vi "GUI_Beampointing2_Pico.vi"() -> ()   [LabVIEW 2020]
uses:
  Shared/GUI_Template/GUI_master/tcp_new_data_event.ctl
  Shared/GUI_Template/GUI_master/tcp new data cluster.ctl
  Ctrs/beam detection.ctl
  Ctrs/move_old.ctl
  Ctrs/stats.ctl
  General GUIs/Device GUIs/GUI_Cameras/Controls/Crosshair type def.ctl
  Ctrs/Motor Calibration.ctl
  <vilib>/Analysis/NI_AALBase.lvlib
panel:
  out "Image":T1(plugin-control)
  in  "size 2":cluster{"xhair size":dbl, "xhair size 2":dbl}={"xhair size"=20.0, "xhair size 2"=20.0} {"xhair size 2" min=0.0 max=0.0; "xhair size" min=0.0 max=0.0}
  in  "Time":timestamp[](array[timestamp])
  in  "Stats 2":T2
  in  "output cluster 2":T3
  in  "UDP error message":string
  in  "Save Stats":bool
  in  "output cluster":T7={"img to avg"=0, "beam detection para"={"Filter"=0, "Filter Para"={"X Size"=0, "Y Size"=0, "% Tolerance"=0}, "detection method"=0, "smal para"=[], "Remove small Objects"=FALSE, "Restrict to round Objects"=FALSE}, "move"={"Tolerance [%]"=0.1, "Stepsize"=0.0001, "Invert Axis"=TRUE, "Invert Direction X"=FALSE, "Invert Direction Y"=TRUE, "enable feedback"=FALSE, "Set Centriod Target"=FALSE, "my active motor"=""}, "GUIdevice 1"="", "GUIdevice 2"="", "ActiveMotor"=0, "stats path "=path ""} {"beam detection para"."smal para"."Measurement Parameter" items=["Center of Mass X", "Center of Mass Y", "First Pixel X", "First Pixel Y", "Bounding Rect Left", "Bounding Rect Top", "Bounding Rect Right", "Bounding Rect Bottom", "Max Feret Diameter Start X", "Max Feret Diameter Start Y", "Max Feret Diameter End X", "Max Feret Diameter End Y", "Max Horiz. Segment Length Left", "Max Horiz. Segment Length Right", "Max Horiz. Segment Length Row", "-", "Bounding Rect Width", "Bounding Rect Height", "Bounding Rect Diagonal", "Perimeter", "Convex Hull Perimeter", "Holes' Perimeter", "Max Feret Diameter", "Equivalent Ellipse Major Axis", "Equivalent Ellipse Minor Axis", "Equivalent Ellipse Minor Axis (Feret)", "Equivalent Rect Long Side", "Equivalent Rect Short Side", "Equivalent Rect Diagonal", "Equivalent Rect Short Side (Feret)", "Average Horiz. Segment Length", "Average Vert. Segment Length", "Hydraulic Radius", "Waddel Disk Diameter", "-", "Area", "Holes' Area", "Particle & Holes' Area", "Convex Hull Area", "Image Area", "-", "Number of Holes", "Number of Horiz. Segments", "Number of Vert. Segments", "-", "Orientation", "Max Feret Diameter Orientation", "-", "% Area/Image Area", "% Area/(Particle & Holes' Area)", "Ratio of Equivalent Ellipse Axes", "Ratio of Equivalent Rect Sides", "-", "Elongation Factor", "Compactness Factor", "Heywood Circularity Factor", "Type Factor", "-", "Sum X", "Sum Y", "Sum XX", "Sum XY", "Sum YY", "Sum XXX", "Sum XXY", "Sum XYY", "Sum YYY", "-", "Moment of Inertia XX", "Moment of Inertia XY", "Moment of Inertia YY", "Moment of Inertia XXX", "Moment of Inertia XXY", "Moment of Inertia XYY", "Moment of Inertia YYY", "Norm. Moment of Inertia XX", "Norm. Moment of Inertia XY", "Norm. Moment of Inertia YY", "Norm. Moment of Inertia XXX", "Norm. Moment of Inertia XXY", "Norm. Moment of Inertia XYY", "Norm. Moment of Inertia YYY", "Hu Moment 1", "Hu Moment 2", "Hu Moment 3", "Hu Moment 4", "Hu Moment 5", "Hu Moment 6", "Hu Moment 7"]; "beam detection para"."smal para"."Range Lower Value" format="%.2f"; "beam detection para"."smal para"."Range Upper Value" format="%.2f"; "beam detection para"."detection method" items=["clustering", "entropy", "metric", "moments", "inter-class variance"]; "beam detection para"."Filter" items=["No Filter", "Median Filter", "Low Pass Filter"]}
  in  "Trigger::1":bool
  in  "Triggerdelay::1":dbl=0.003 min=0.0 max=50000.0 format="%#_6f"
  in  "Exposure::1":dbl=0.095 min=0.0001 max=1.0 format="%#_6f"
  in  "ActiveMotorName::2":string
  in  "RelativeSettings.Axis 1.StepSize::2":dbl=50.0 caption="Axis 1 Stepsize" min=0.0 max=999999.0 format="%_4p"
  in  "RelativeSettings.Axis 2.StepSize::2":dbl=50.0 caption="Axis 2 StepSize" min=0.0 max=999999.0 format="%_4p"
  in  "RelativeSettings.Axis 2.Position::2":dbl caption="Axis 2 Position" min=-999999.0 max=999999.0 format="%_4p"
  in  "RelativeSettings.Axis 1.Position::2":dbl caption="Axis 1 Position" min=-999999.0 max=999999.0 format="%_4p"
  in  "RelativeMove.Axis 2.CW::2":bool caption="RelativeMove.Axis 2.CW::1"
  in  "RelativeMove.Axis 2.CCW::2":bool caption="RelativeMove.Axis. 2.CCW::1"
  in  "RelativeMove.Axis 1.CW::2":bool caption="RelativeMove.Axis 1.CW::1"
  in  "RelativeMove.Axis 1.CCW::2":bool caption="RelativeMove.Axis 1.CCW::1"
  out "Names":string[](array[string])=["PA2_Input1", "PA2_Input2", "L2_TelInpFar", "L1_TelInpNear", "L4_TREXPASS1", "L5_TREXPass2", "L6_TREXPass3", "L7_TREXPass4", "L8_M10Leak", "B1_TelInput", "B2_TelLens1"]
  in  "ActiveMotor":u16(ring)=7 items=["PA2_Input1", "PA2_Input2", "L2_TelInpFar", "L1_TelInpNear"]
  in  "Set Centriod Target":bool
  in  "size":dbl=10.299999999999997
  in  "Tab Control 2":enum32{"CCD Original ", "CCD Detected"}(tab)=enum."CCD Detected"
  out "image::1":T1(plugin-control) caption="StagingM1Far"
  out "Beam":T1(plugin-control)
  in  "Reset History":bool
  out "centriod X":dbl[](graph)=[249.59745762711864, 249.9873417721519, 249.85593220338984]
  out "centriod Y":dbl[](graph)=[256.39830508474574, 256.0126582278481, 257.0]
  out "Stats":cluster{timestamp[], dbl[]}[](graph)
  in  "Tab Control":enum32{"System", "Detection", "Feedback"}(tab)=enum."Feedback"
  in  "Save Stats":bool
  in  "update speed [ms]":i32=200
  in  "img to avg":i32=20
  in  "Save Config":bool
  in  "Load Config":bool
  in  "Cameras":u16(ring)=15 items=["10TW_Driver_Spot_Cam", "B1_TelInput", "B2_TelLens1", "B3_TelLens2", "B5_CompressorOut", "B6_SwitchYNear", "B9_OAPFront", "GIGEtest", "L1_TelInpNear", "L2_TelInpFar", "L3_TelescopeOut", "L4_TREXpass1", "L5_TREXPass2", "L6_TREXpass3", "L7_TREXPass4", "L8_M10Leak", "OAPtestCam", "PA2_Input1", "PA2_Input2", "PaperCam", "StagingAlignBeam1", "StagingAlignBeam2", "StagingCapAlignment", "StagingCapSpec", "StagingCapSpec1stOrder", "StagingChromaxGuppy", "StagingDiodeMonitor", "StagingFocusBeam1", "StagingFocusBeam2", "StagingGuppy", "StagingM1Far", "StagingM1Near", "StagingM3Far", "StagingM4", "StagingM5", "StagingMagnetCam1", "StagingMagnetCam2", "StagingMagnetCam3", "StagingManta2", "StagingModeImager2", "StagingModeTemp", "StagingOAP1Far", "StagingOAP1Near", "StagingOAP2Far", "StagingOAP2Near", "StagingPhasics", "StagingPhosphor", "StagingTapeCam", "StagingTapeMonitorCam", "StagingTopView", "TargetCam10Hz_Diode", "TargetCam1Hz_Pulsed", "TREXVarianCam0", "TREXVarianCam1", "TREXVarianCam2", "TREXVarianCam3", "TREX_CapSideView", "TREX_TA6", "TS-253a_in", "TS-CapSideview", "TS-CapSpec", "TS-ChromexCam", "TS-InputNearField", "TS-Mode1", "TS-OverlapCam", "TS-Periscope", "XUV_Cam1", "XUV_Cam2"]
  in  "calibrate":bool
  in  "stats path":path
  in  "beam detection para":T4={"Filter"=1, "Filter Para"={"X Size"=5, "Y Size"=5, "% Tolerance"=1}, "detection method"=4, "smal para"=[{"Measurement Parameter"=35, "Range Lower Value"=150.0, "Range Upper Value"=300.0, "Range"=FALSE, "Measurement Type"=FALSE}], "Remove small Objects"=TRUE, "Restrict to round Objects"=FALSE} {"smal para"."Measurement Parameter" items=["Center of Mass X", "Center of Mass Y", "First Pixel X", "First Pixel Y", "Bounding Rect Left", "Bounding Rect Top", "Bounding Rect Right", "Bounding Rect Bottom", "Max Feret Diameter Start X", "Max Feret Diameter Start Y", "Max Feret Diameter End X", "Max Feret Diameter End Y", "Max Horiz. Segment Length Left", "Max Horiz. Segment Length Right", "Max Horiz. Segment Length Row", "-", "Bounding Rect Width", "Bounding Rect Height", "Bounding Rect Diagonal", "Perimeter", "Convex Hull Perimeter", "Holes' Perimeter", "Max Feret Diameter", "Equivalent Ellipse Major Axis", "Equivalent Ellipse Minor Axis", "Equivalent Ellipse Minor Axis (Feret)", "Equivalent Rect Long Side", "Equivalent Rect Short Side", "Equivalent Rect Diagonal", "Equivalent Rect Short Side (Feret)", "Average Horiz. Segment Length", "Average Vert. Segment Length", "Hydraulic Radius", "Waddel Disk Diameter", "-", "Area", "Holes' Area", "Particle & Holes' Area", "Convex Hull Area", "Image Area", "-", "Number of Holes", "Number of Horiz. Segments", "Number of Vert. Segments", "-", "Orientation", "Max Feret Diameter Orientation", "-", "% Area/Image Area", "% Area/(Particle & Holes' Area)", "Ratio of Equivalent Ellipse Axes", "Ratio of Equivalent Rect Sides", "-", "Elongation Factor", "Compactness Factor", "Heywood Circularity Factor", "Type Factor", "-", "Sum X", "Sum Y", "Sum XX", "Sum XY", "Sum YY", "Sum XXX", "Sum XXY", "Sum XYY", "Sum YYY", "-", "Moment of Inertia XX", "Moment of Inertia XY", "Moment of Inertia YY", "Moment of Inertia XXX", "Moment of Inertia XXY", "Moment of Inertia XYY", "Moment of Inertia YYY", "Norm. Moment of Inertia XX", "Norm. Moment of Inertia XY", "Norm. Moment of Inertia YY", "Norm. Moment of Inertia XXX", "Norm. Moment of Inertia XXY", "Norm. Moment of Inertia XYY", "Norm. Moment of Inertia YYY", "Hu Moment 1", "Hu Moment 2", "Hu Moment 3", "Hu Moment 4", "Hu Moment 5", "Hu Moment 6", "Hu Moment 7"]; "smal para"."Range Lower Value" format="%.2f"; "smal para"."Range Upper Value" format="%.2f"; "detection method" items=["clustering", "entropy", "metric", "moments", "inter-class variance"]; "Filter" items=["No Filter", "Median Filter", "Low Pass Filter"]}
  in  "Move Properties":T6={"Tolerance [%]"=0.1, "Stepsize"=0.0001, "Invert Axis"=TRUE, "Invert Direction X"=FALSE, "Invert Direction Y"=TRUE, "enable feedback"=FALSE, "Set Centriod Target"=FALSE, "my active motor"=""} {"Stepsize" format="%#_6p"}
  out "Y Size":dbl=20.599999999999994
  out "X Size":dbl=15.599999999999994
  out "Particle Reports (Pixels)":T8(array[cluster])=[{"Area"=236.0, "Number of Holes"=0.0, "Bounding Rect"={"Left"=243.0, "Top"=247.0, "Right"=258.0, "Bottom"=268.0}, "Center of Mass"={"X"=249.85593220338984, "Y"=257.0}, "Orientation"=87.89795034558499, "Dimensions"={"Width"=15.0, "Height"=21.0}}] {"Orientation" format="%.2f"; "Dimensions"."Height" format="%.2f"; "Dimensions"."Width" format="%.2f"; "Center of Mass"."Y" format="%.2f"; "Center of Mass"."X" format="%.2f"; "Bounding Rect"."Bottom" format="%.2f"; "Bounding Rect"."Right" format="%.2f"; "Bounding Rect"."Top" format="%.2f"; "Bounding Rect"."Left" format="%.2f"; "Number of Holes" format="%.2f"; "Area" format="%.2f"}
  out "move required":bool=TRUE
  out "moving":bool
  out "Best Rectangle":T9(array[cluster])=[{"Left"=243.0, "Top"=247.0, "Right"=259.0, "Bottom"=267.0}, {"Left"=242.0, "Top"=246.0, "Right"=257.0, "Bottom"=267.0}, {"Left"=242.0, "Top"=246.0, "Right"=258.0, "Bottom"=267.0}, {"Left"=243.0, "Top"=247.0, "Right"=258.0, "Bottom"=268.0}, {"Left"=242.0, "Top"=247.0, "Right"=258.0, "Bottom"=267.0}]
  out "XY Graph":cluster{timestamp[], dbl[]}[](graph)
  out "Y offset":dbl=-1.5635377104373447
  out "X offset":dbl=10.405838585398385
  in  "Target.X::1":dbl=260.0 min=0.0 max=2000.0 format="%#_6f"
  in  "Target.Y::1":dbl=255.0 min=0.0 max=2000.0 format="%#_6f"
  out "mean Y":dbl=256.56353771043734 format="%0.2f"
  out "mean X":dbl=249.59416141460161 format="%0.2f"
  out "beam detected":bool=TRUE
  in  "GUIdevice 2":string="Picopad4"
  out "error out":errorcluster
  in  "insert tag":bool=TRUE
  in  "stop":bool=TRUE
  in  "GUIdevice 1":string="B5_CompressorOut"
  out "tcp data event":T10
  out "error IO 2":errorcluster
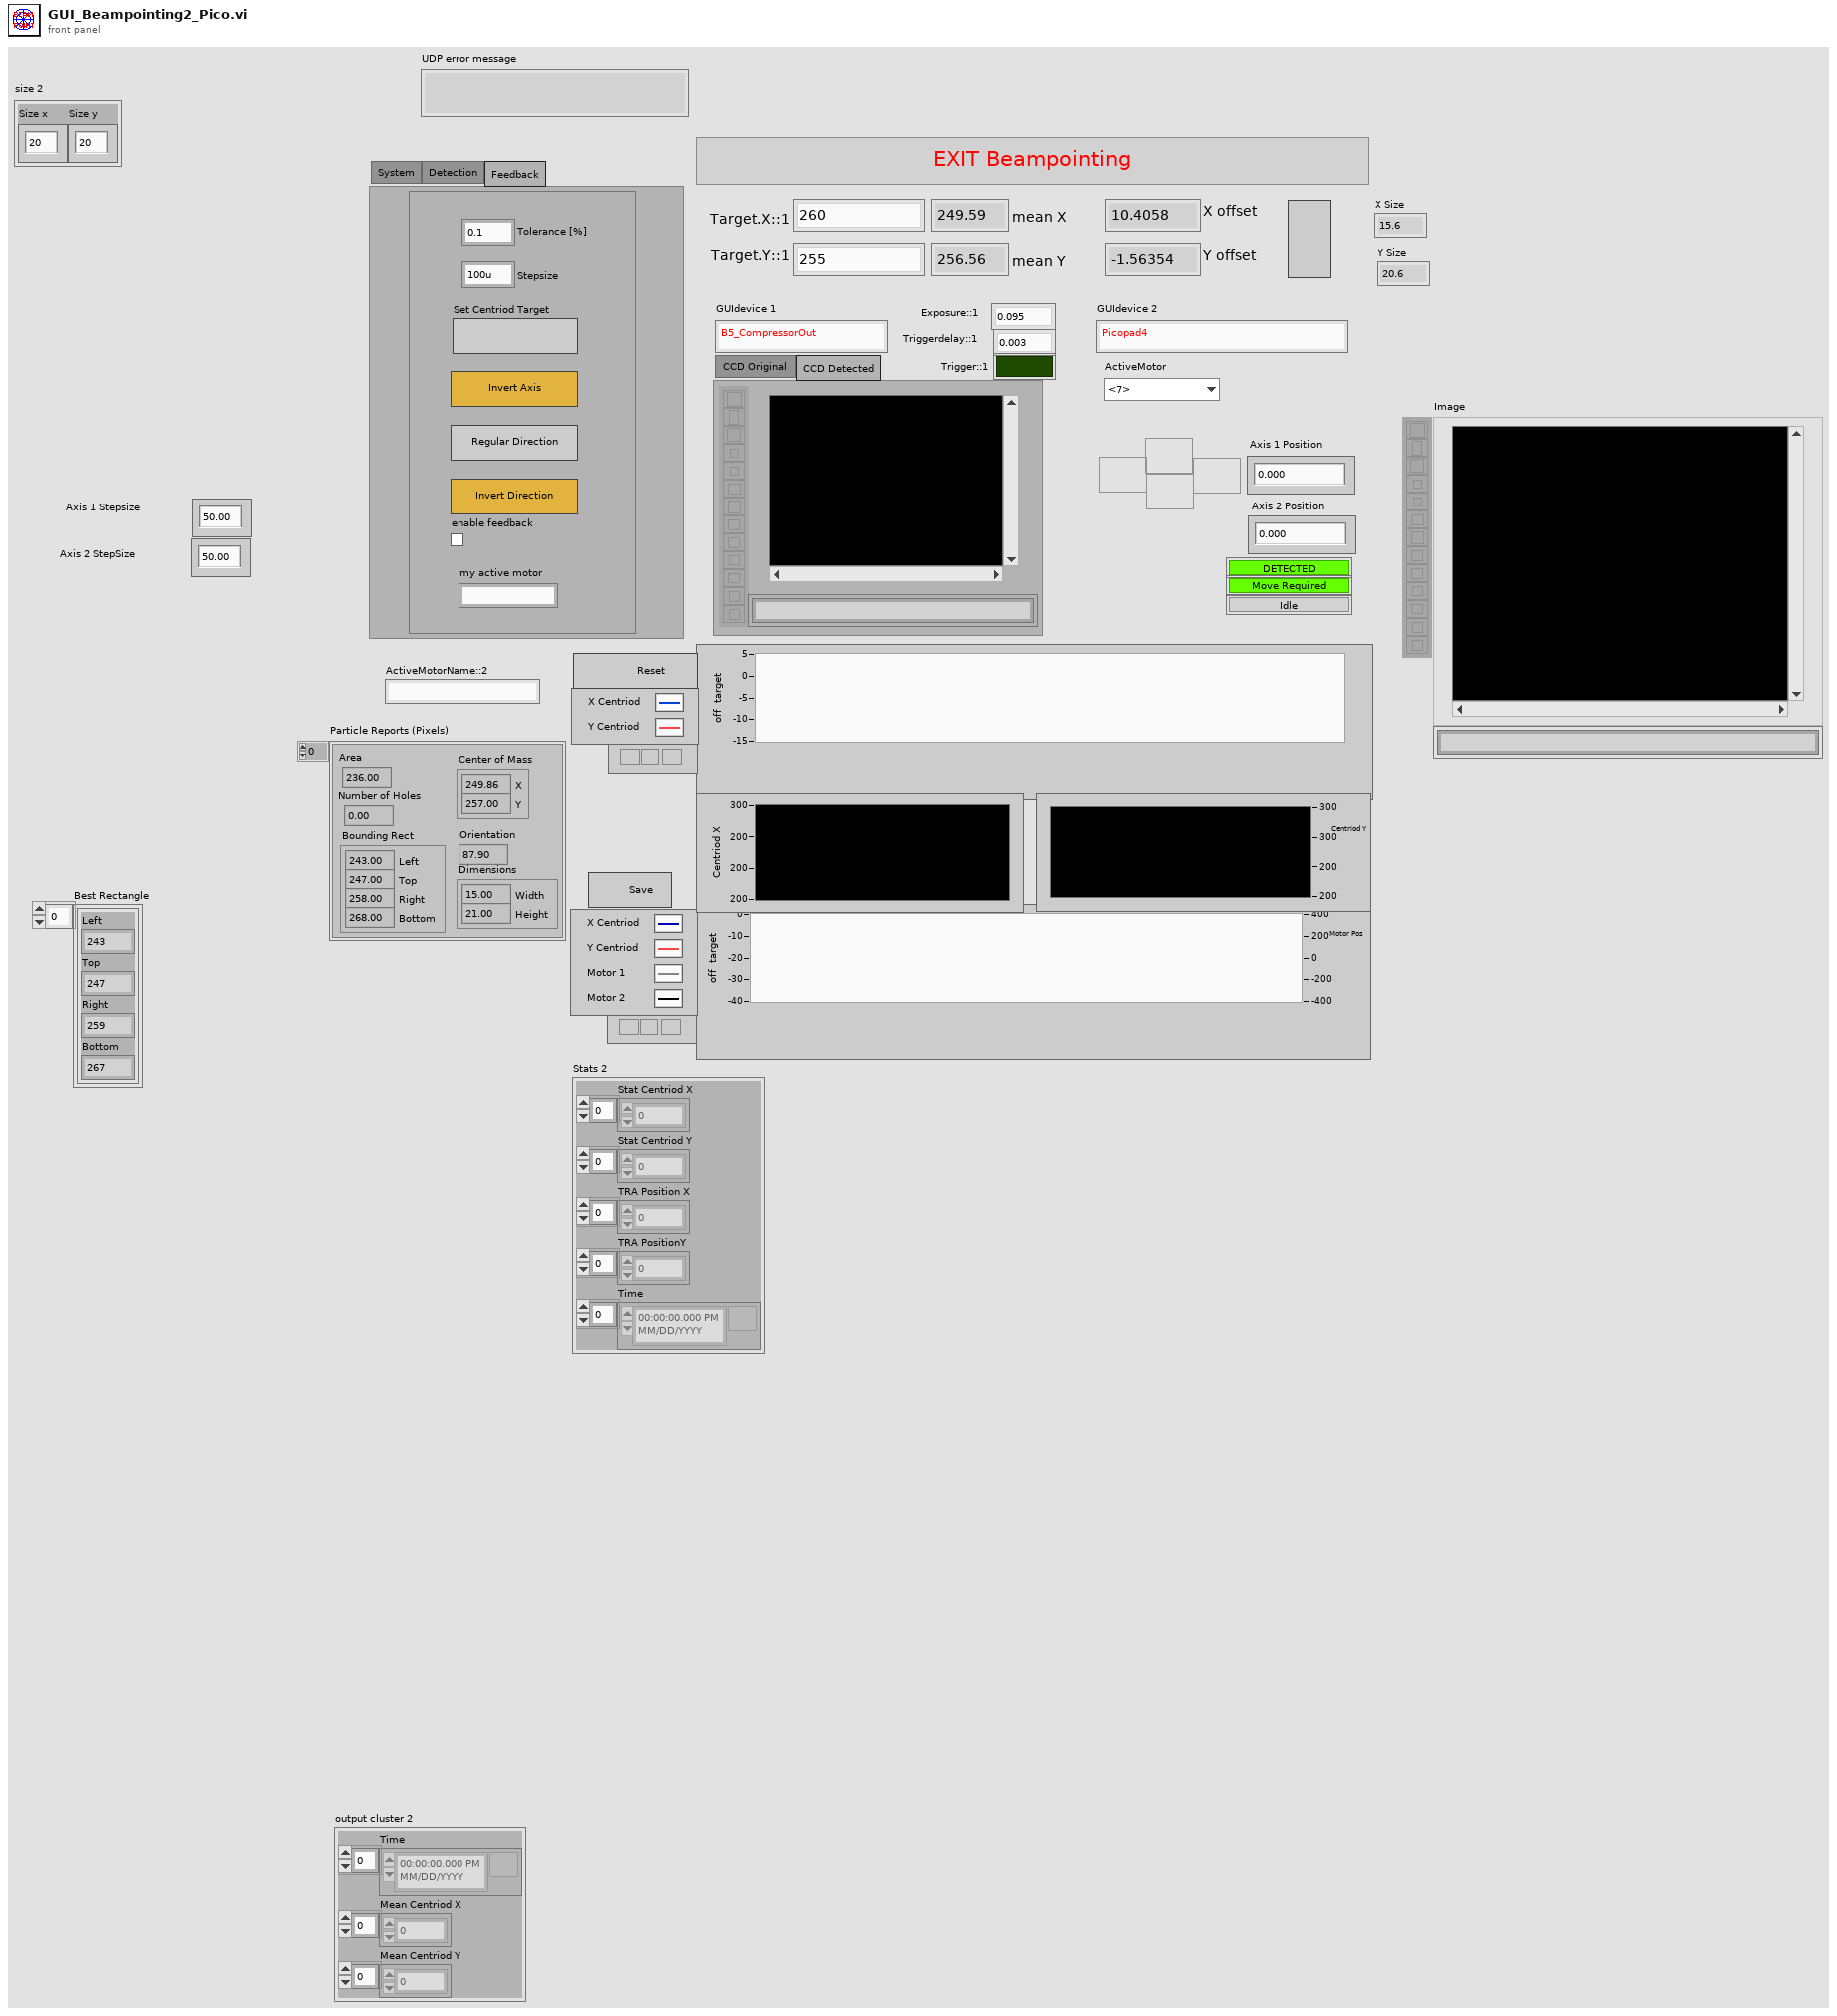
[diagram p1: front panel]
types:
  T1 = typedef "IMAQ Image.ctl" = refnum<image>
  T2 = typedef "stats.ctl" = cluster{"Stat Centriod X":dbl[], "Stat Centriod Y":dbl[], "TRA Position X":dbl[], "TRA PositionY":dbl[], "Time":timestamp[]}
  T3 = cluster{"Time":timestamp[], "Mean Centriod X":dbl[], "Mean Centriod Y":dbl[]}
  T4 = typedef "beam detection.ctl" = cluster{"Filter":u16, "Filter Para":cluster{"X Size":i32, "Y Size":i32, "% Tolerance":i32}, "detection method":i32, "smal para":cluster{"Measurement Parameter":T5, "Range Lower Value":dbl, "Range Upper Value":dbl, "Range":bool, "Measurement Type":bool}[], "Remove small Objects":bool, "Restrict to round Objects":bool}
  T5 = typedef "Particle Parameters" = i32
  T6 = typedef "move_old.ctl" = cluster{"Tolerance [%]":dbl, "Stepsize":dbl, "Invert Axis":bool, "Invert Direction X":bool, "Invert Direction Y":bool, "enable feedback":bool, "Set Centriod Target":bool, "my active motor":string}
  T7 = cluster{"img to avg":i32, "beam detection para":T4, "move":T6, "GUIdevice 1":string, "GUIdevice 2":string, "ActiveMotor":u16, "stats path ":path}
  T8 = cluster{"Area":dbl, "Number of Holes":dbl, "Bounding Rect":cluster{"Left":dbl, "Top":dbl, "Right":dbl, "Bottom":dbl}, "Center of Mass":cluster{"X":dbl, "Y":dbl}, "Orientation":dbl, "Dimensions":cluster{"Width":dbl, "Height":dbl}}[]
  T9 = cluster{"Left":dbl, "Top":dbl, "Right":dbl, "Bottom":dbl}[]
  T10 = typedef "tcp_new_data_event.ctl" = refnum<user-event>
  T11 = typedef "tcp new data cluster.ctl" = cluster{"EventEnum":enum16{"new data", "connection status update"}, "Device name":string}
  T12 = typedef "Image Type" = u32
  T13 = cluster{"RelativeMove.Axis 1.CW::2":refnum<vi>, "RelativeMove.Axis 1.CCW::2":refnum<vi>, "RelativeMove.Axis 2.CW::2":refnum<vi>, "RelativeMove.Axis 2.CCW::2":refnum<vi>}
  T14 = typedef "Crosshair type def.ctl" = cluster{"Draw":bool, "Target":cluster{"x":dbl, "y":dbl}, "Size":cluster{"x":dbl, "y":dbl}, "Angle":dbl, "Color":u32, "Thickness":u8, "CrosshairLabel":string}
  T15 = cluster{"Left":i32, "Top":i32, "Right":i32, "Bottom":i32}
  T16 = enum32{"invalid app kind", "Development System", "Run Time System", "Student Edition", "Embedded LabVIEW", "Evaluation", "Custom"}
  T17 = enum32{"Invalid", "Standard", "Closed", "Hidden", "Minimized", "Maximized"}
  T18 = enum16{"open", "replace", "create", "open or create", "replace or create", "replace or create with confirmation"}
  T19 = typedef "Motor Calibration.ctl" = cluster{"Slope Axis 1":dbl, "Axis Inverted":bool, "Slope Axis 2":dbl, "Axis 1 revered":bool, "Axis 2 revered":bool}
  T20 = cluster{"Core":cluster{"Current VI Reference":refnum<vi>, "Close Panel on Exit?":bool}, "beam detection para":T4, "Centriod X":dbl[], "Centriod Y":dbl[], "Best Rectangle":cluster{"Left":dbl, "Top":dbl, "Right":dbl, "Bottom":dbl}[], "PArticle Report":cluster{"Area":dbl, "Number of Holes":dbl, "Bounding Rect":cluster{"Left":dbl, "Top":dbl, "Right":dbl, "Bottom":dbl}, "Center of Mass":cluster{"X":dbl, "Y":dbl}, "Orientation":dbl, "Dimensions":cluster{"Width":dbl, "Height":dbl}}[], "Mean Centriod X":dbl[], "Mean Centriod Y":dbl[], "Time":timestamp[], "beam detected":bool, "offsets":cluster{"X offset":dbl, "Y offset":dbl}, "move":T6, "moving":bool, "Stats":T2, "set centriod target":bool, "Motor Calibration":T19}
  T21 = cluster{"Left":dbl, "Top":dbl, "Right":dbl, "Bottom":dbl}
  T22 = cluster{"Current VI Reference":refnum<vi>, "Close Panel on Exit?":bool}
  T23 = cluster{"Time":timestamp[], "Stat Centriod X":dbl[]}
  T24 = cluster{"Time":timestamp[], "Stat Centriod Y":dbl[]}
  T25 = cluster{"Time":timestamp[], "TRA Position X":dbl[]}
  T26 = cluster{"Time":timestamp[], "TRA PositionY":dbl[]}
  T27 = cluster{"Time":timestamp[], "TRA PositionY":dbl[]}[]
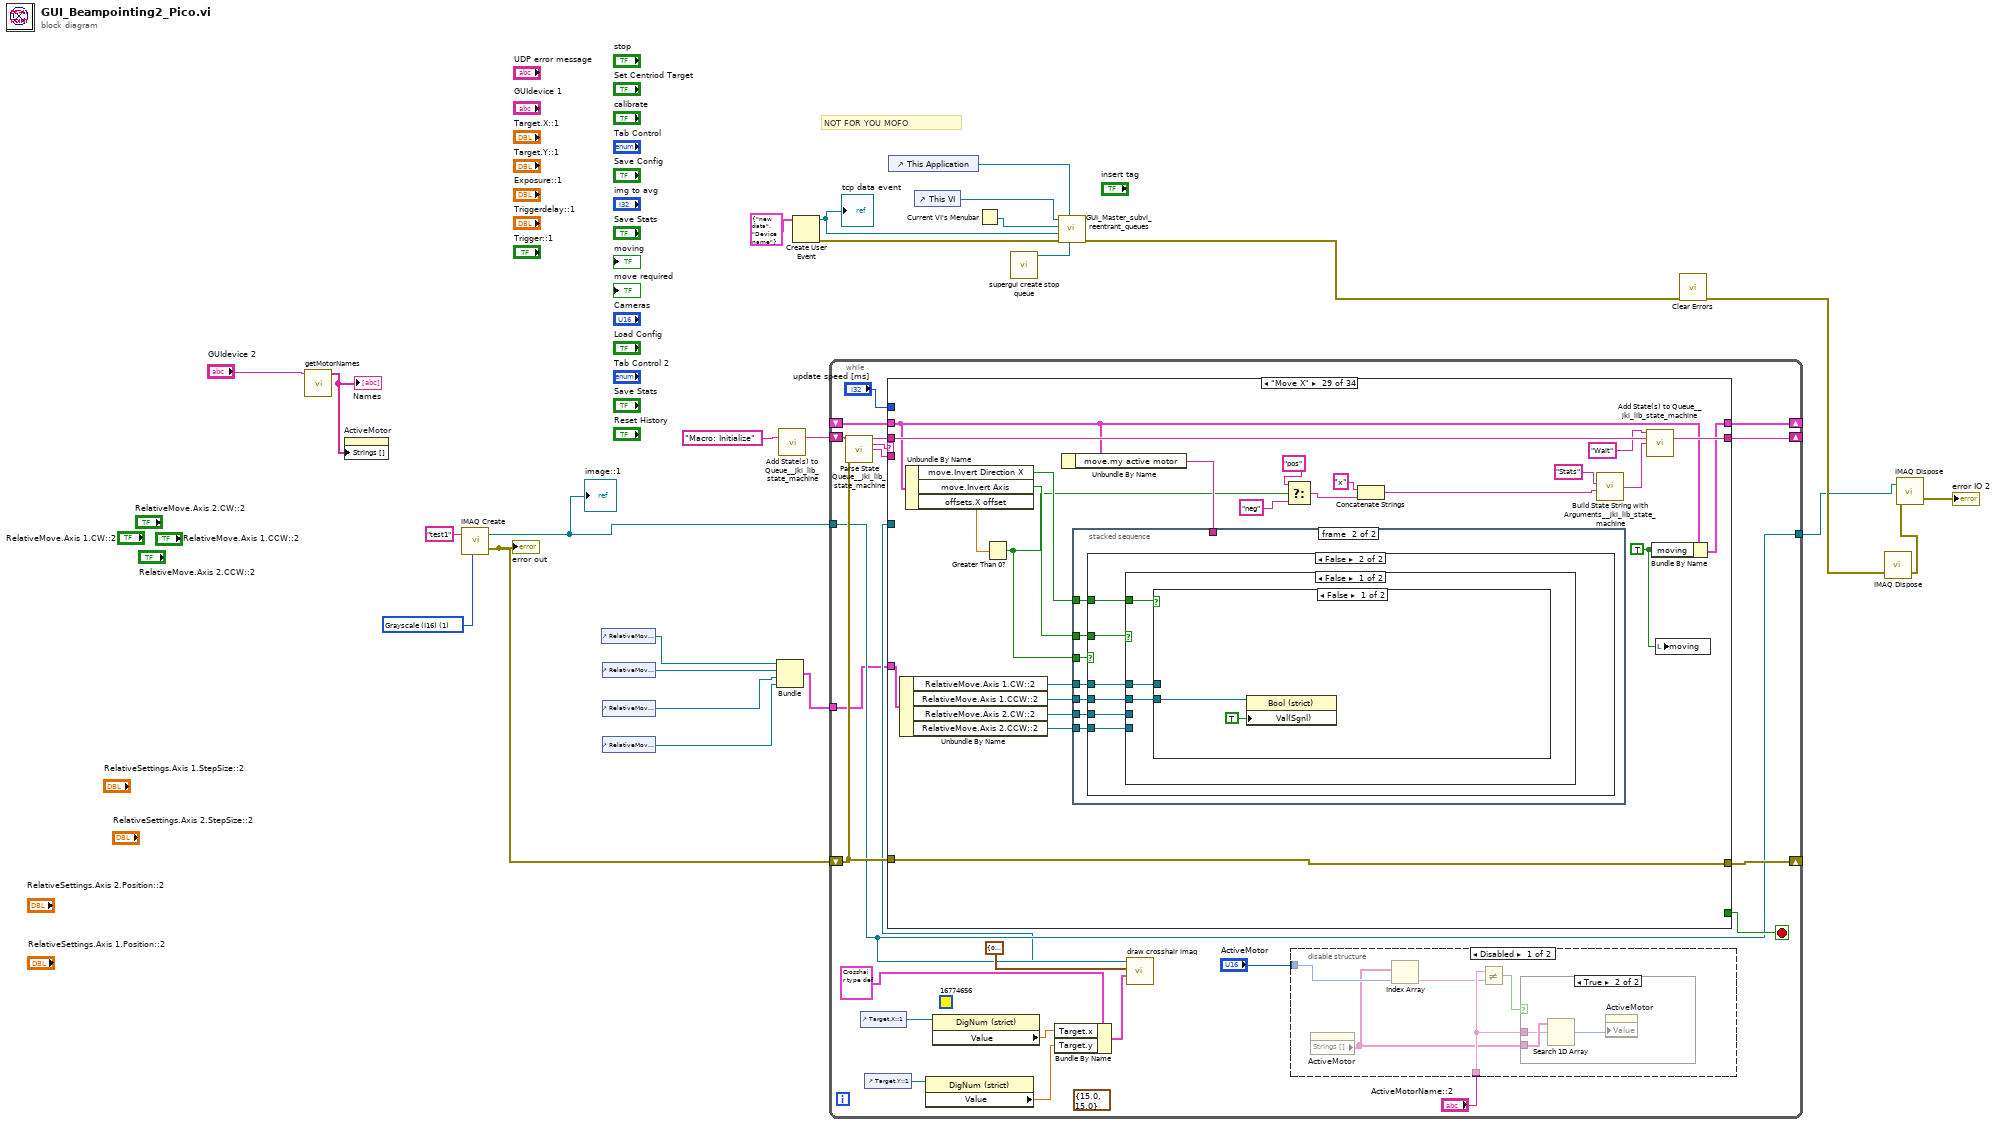
[diagram p0: block diagram]
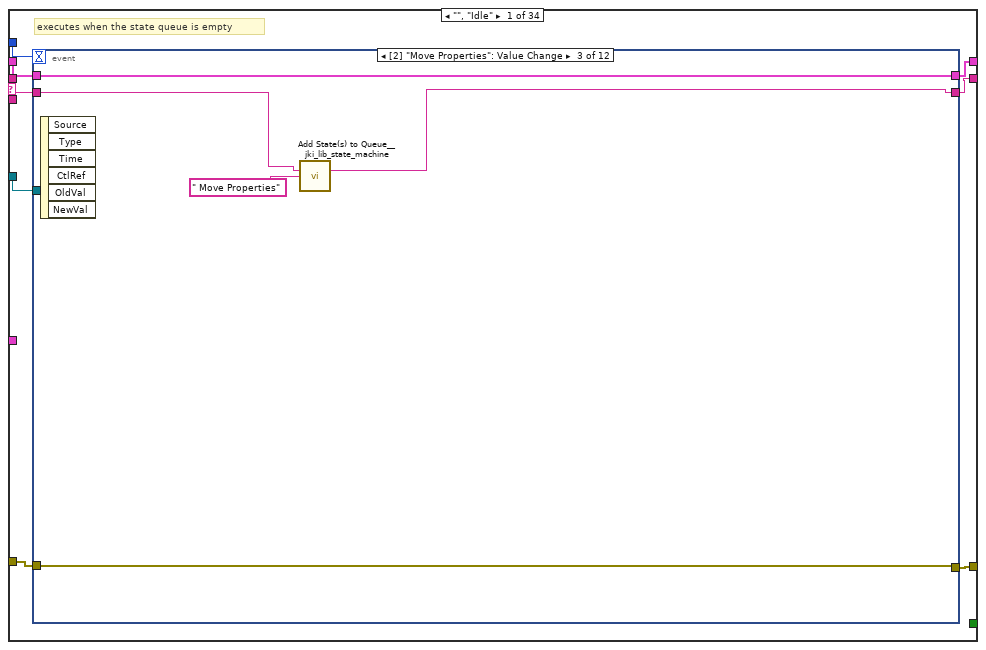
[diagram p4: hidden frame]
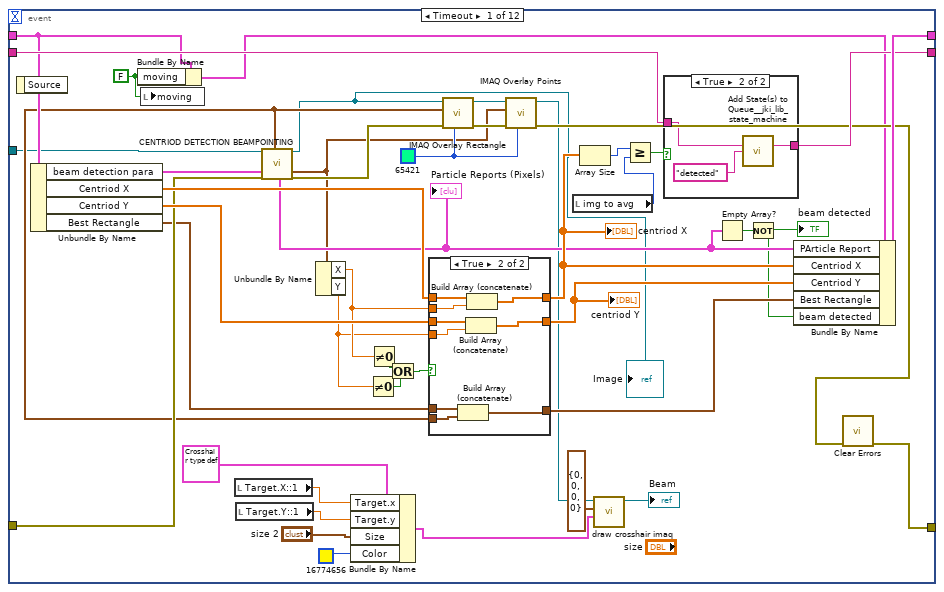
[diagram p5: hidden frame]
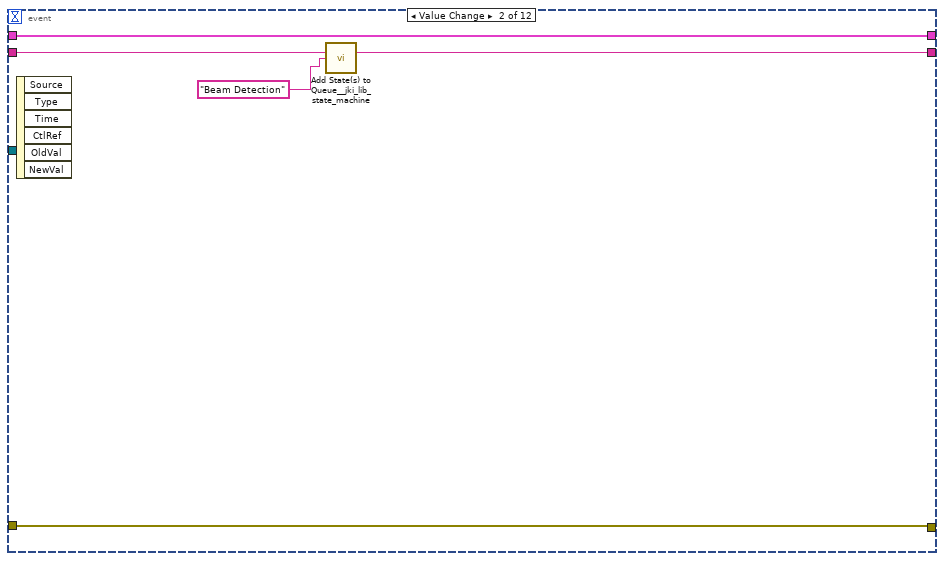
[diagram p8: hidden frame]
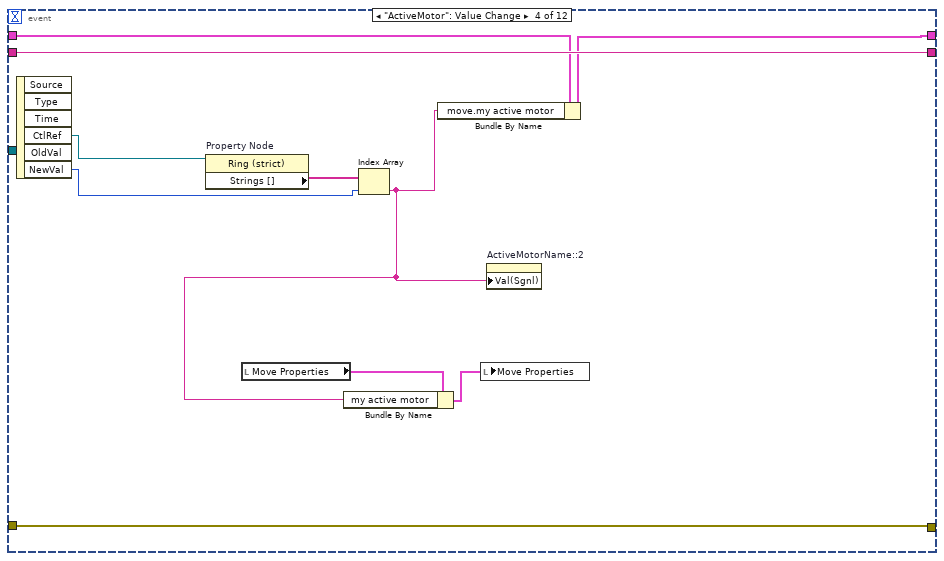
[diagram p9: hidden frame]
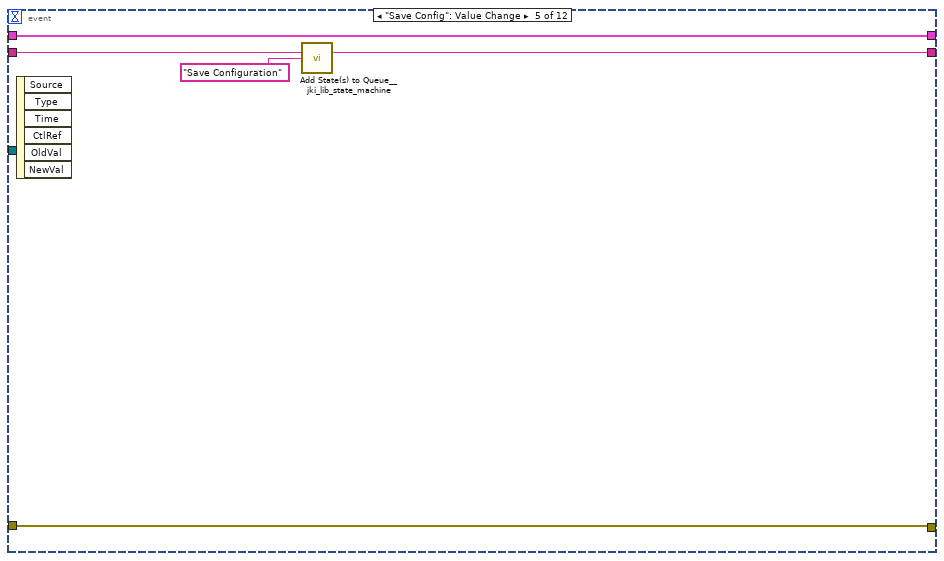
[diagram p10: hidden frame]
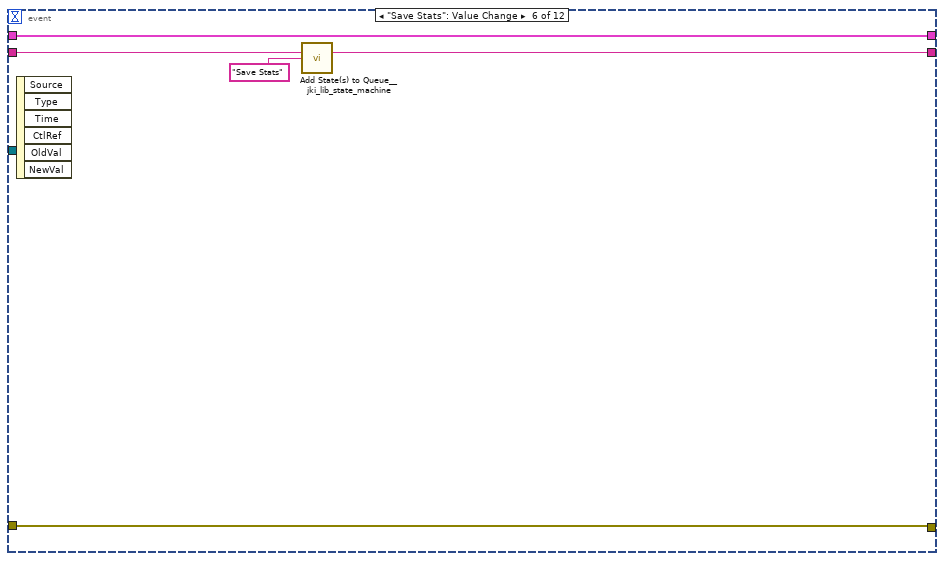
[diagram p11: hidden frame]
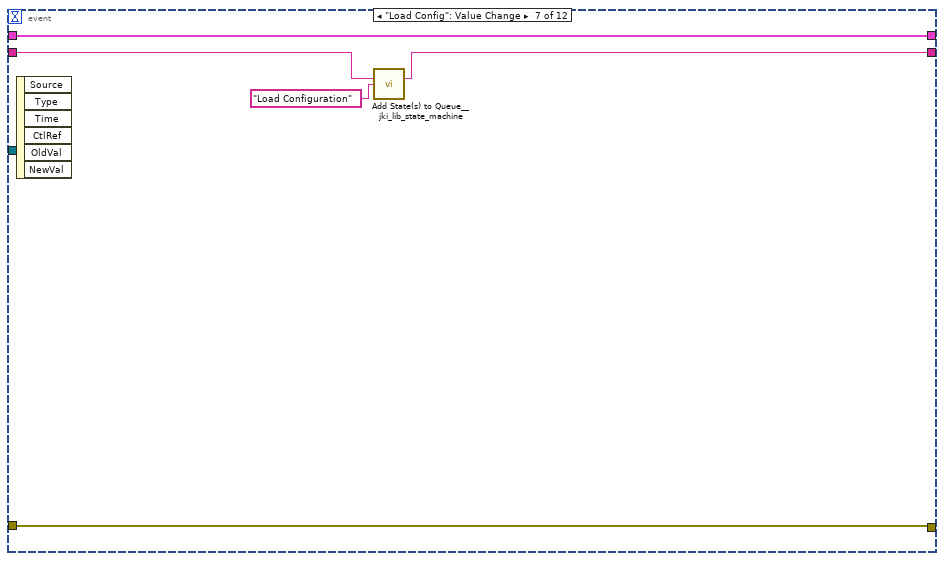
[diagram p12: hidden frame]
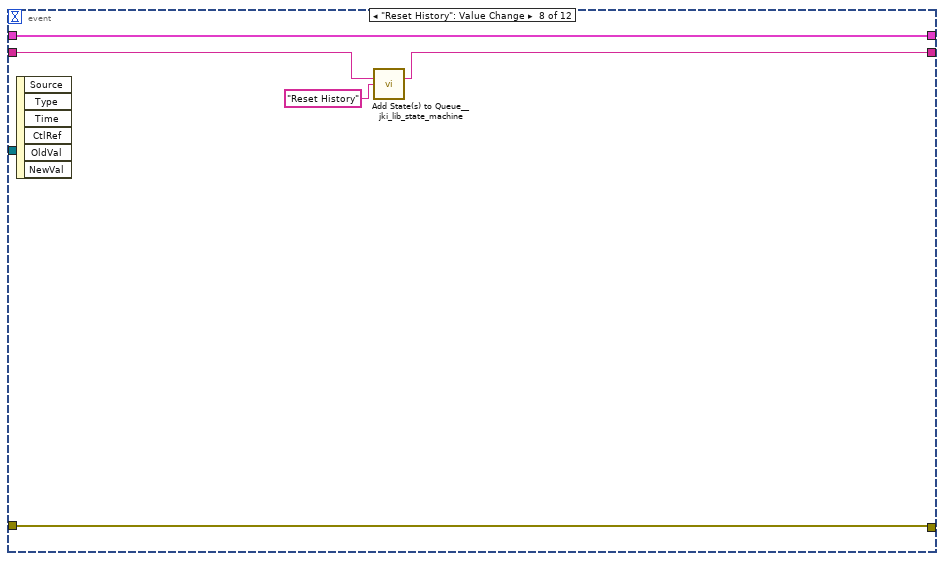
[diagram p13: hidden frame]
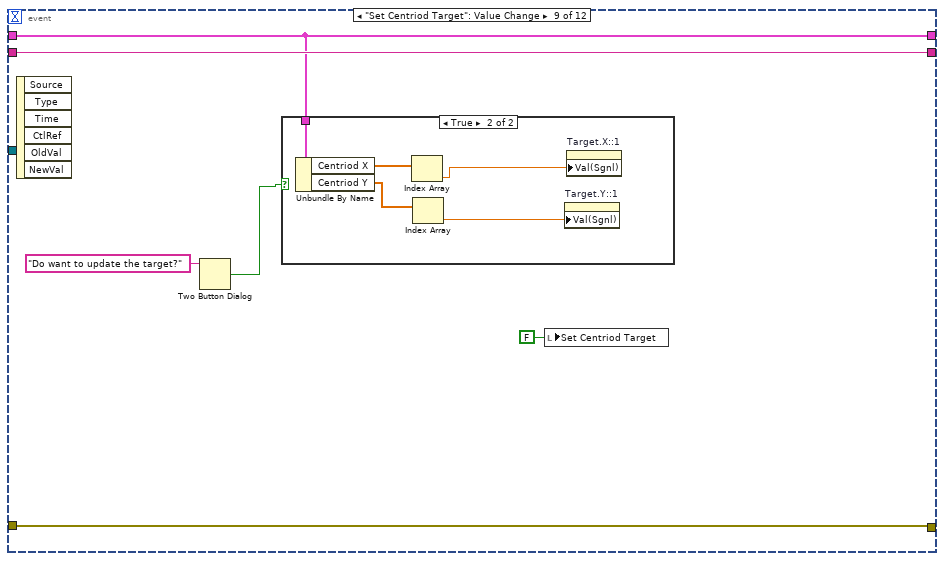
[diagram p14: hidden frame]
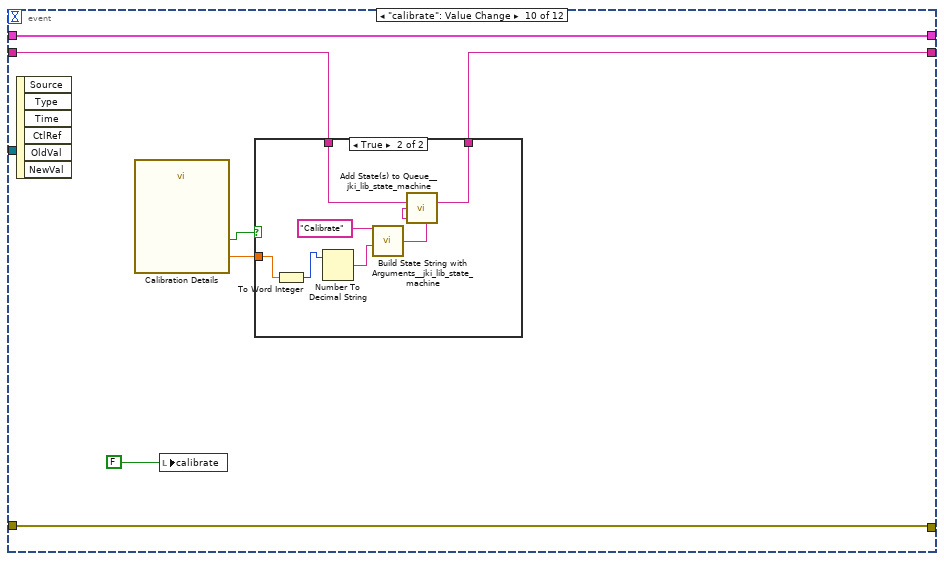
[diagram p16: hidden frame]
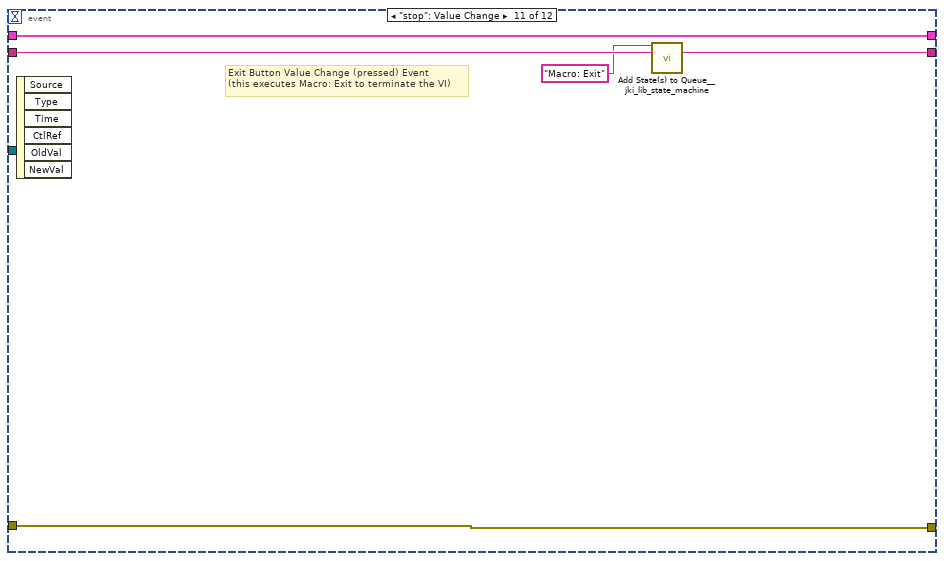
[diagram p18: hidden frame]
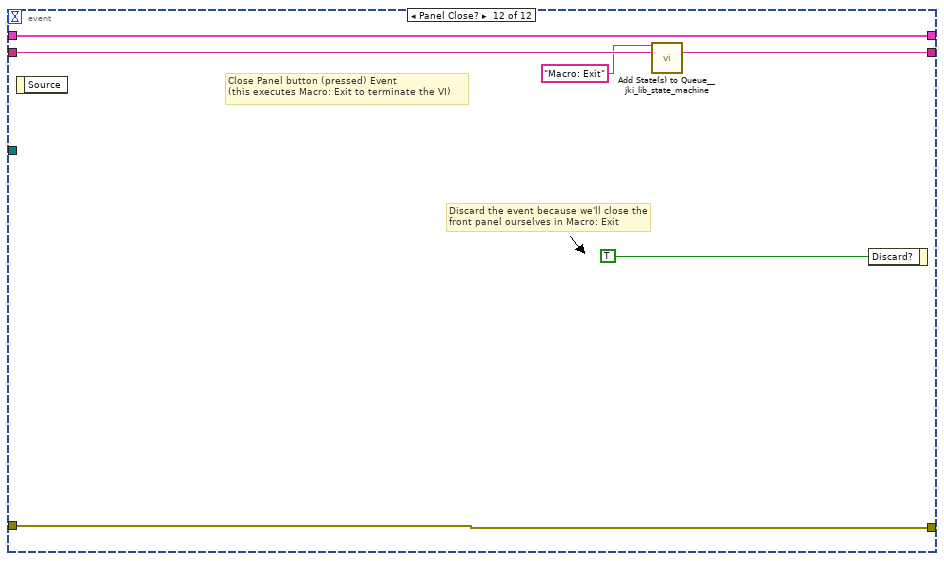
[diagram p19: hidden frame]
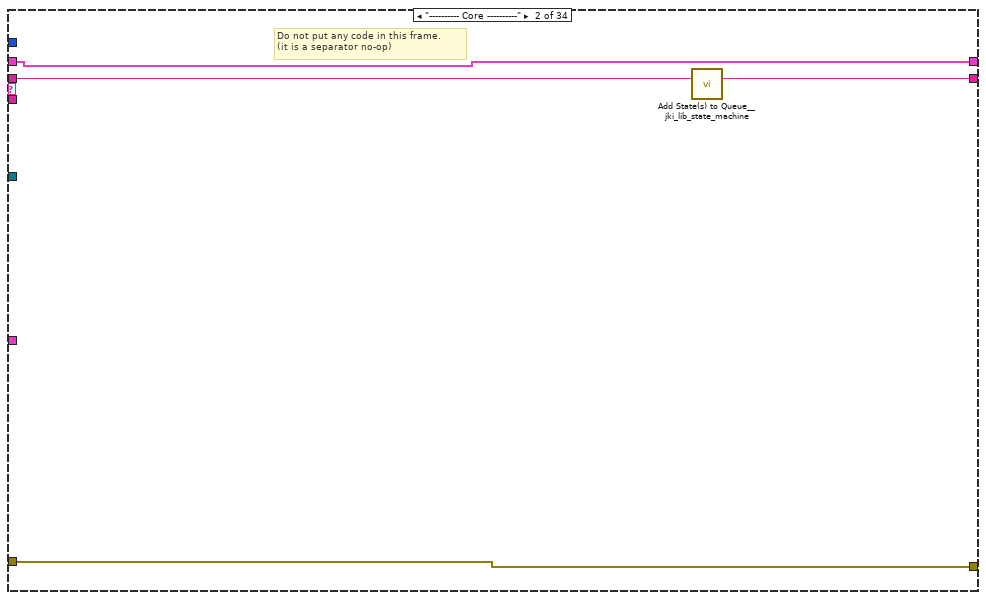
[diagram p20: hidden frame]
diagram:
  w24 = T12 1 items=["Grayscale (U8)", "Grayscale (I16)", "Grayscale (SGL)", "Complex (CSG)", "RGB (U32)", "HSL (U32)", "RGB (U64)", "Grayscale (U16)"] ("Image Type")
  # "NOT FOR YOU MOFO"
  n1 = call "getMotorNames.vi"("DeviceName"="GUIdevice 2") -> ("elements"=w7:string[])  [unwired: 10 in]
  "Names" <- w7
  n2 = property on="ActiveMotor" class="Ring (strict)"("Strings []"=w7) -> ()  [unwired: 2 in, 2 out]
  n3 = call "IMAQ Create"("Image Name"="test1", "Image Type"=w24) -> ("New Image"=w9:T1, "error out"=w17:errorcluster)  [unwired: 3 in]
  "error out" <- w17
  "image::1" <- w9
  n4 = control-ref of="RelativeMove.Axis 1.CW::2"() -> (w6:refnum<vi>)
  n5 = control-ref of="RelativeMove.Axis 1.CCW::2"() -> (w5:refnum<vi>)
  n6 = control-ref of="RelativeMove.Axis 2.CW::2"() -> (w4:refnum<vi>)
  n7 = control-ref of="RelativeMove.Axis 2.CCW::2"() -> (w3:refnum<vi>)
  n8 = Bundle("RelativeMove.Axis 1.CW::2"=w6, "RelativeMove.Axis 1.CCW::2"=w5, "RelativeMove.Axis 2.CW::2"=w4, "RelativeMove.Axis 2.CCW::2"=w3) -> (w2:T13)  [unwired: 1 in]
  n9 = call <vilib>:"Add State(s) to Queue__jki_lib_state_machine.vi"("State(s) in (\"\")"="Macro: Initialize") -> ("States Out"=w19:string)  [unwired: 14 in]
  n10 = Create User Event(user event datatype=T11 {"EventEnum"=enum."new data", "Device name"="Device name"} ("New Event")) -> (user event=w10:refnum<user-event>, error out=w12:errorcluster)  [unwired: 1 in]
  "tcp data event" <- w10
  n11 = while "JKI - String-Based Queued State Machine (Basic) v1.0" {
    shift-right: [w42] -> _
    shift-left: _ -> [w41]
    shift-right: [w44] -> _
    shift-left: w17 -> [w39]
    shift-right: [w43] -> _
    shift-left: w19 -> [w45]
    tunnel: w9 -> [w34]
    tunnel: [w34] -> w16
    tunnel: w2 -> [w32]
    stop <- w38 stop-if-true
    (unwired) cluster{"xhair size":dbl, "xhair size 2":dbl} {"xhair size"=15.0, "xhair size 2"=15.0} ("size")
    (unwired) u32 16774656 ("Color")
    n12 = call <vilib>:"Parse State Queue__jki_lib_state_machine.vi"("State Queue"=w45, "Error In (no error)"=w39) -> ("Remaining States"=w47:string, "Current State"=w48:string, "Arguments"=w46:string)  [unwired: 11 in]
    n13 = control-ref of="Target.X::1"() -> (w36:refnum<vi>)
    n14 = control-ref of="Target.Y::1"() -> (w37:refnum<vi>)
    n15 = property class="DigNum (strict)"(reference=w37) -> ("Value"=w27:dbl)  [unwired: 1 in, 2 out]
    n16 = property class="DigNum (strict)"(reference=w36) -> ("Value"=w28:dbl)  [unwired: 1 in, 2 out]
    n17 = Bundle By Name(cluster=T14 {"Draw"=TRUE, "Target"={"x"=25.0, "y"=25.0}, "Size"={"x"=25.0, "y"=25.0}, "Angle"=0.0, "Color"=8322834, "Thickness"=1, "CrosshairLabel"=""} ("Crosshair"), "Target.x"=w28, "Target.y"=w27) -> (w26:T14)
    n18 = call "draw crosshair imaq.vi"("Crosshair"=w26, "Bounding Rectangle"=T15 {"Left"=0, "Top"=0, "Right"=0, "Bottom"=0}, "image in"=w34) -> ("image out"=w33:T1)  [unwired: 7 in, 1 out]
    n19 = case shown="\"Move X\"" w48 {
      selector: w48 -> [_ _ w206 _ _ _ _ _ _ _ _ _ _ _ _ _ _ _ _ _ _ _ _ _ _ _ _ _ _ _ _ _ _ _]
      tunnel: w47 -> [w64 w205 w210 w228 w234 w239 w243 w267 w273 w277 w281 w287 w298 w324 w329 w339 w343 w349 w356 w377 w385 w406 w442 w450 w454 w487 w497 w534 w558 w630 w690 w703 w778 w782]
      tunnel: w46 -> [_ _ _ _ _ _ _ _ _ _ _ w282 w292 _ _ _ _ _ _ _ _ _ _ _ _ _ _ _ _ _ _ w696 w773 _]
      tunnel: w41 -> [w62 w202 w208 w219 w231 w237 w240 _ w269 w274 w279 w285 w294 w321 w326 w336 w340 w345 w352 w360 w383 w404 w434 w446 w451 w470 w499 w531 w545 w617 w686 w725 w775 w779]
      tunnel: [w61 w203 w212 w225 errorcluster {"status"=FALSE, "code"=0, "source"=""} ("error out") w236 w241 w264 w270 w275 w278 w283 w295 w322 w327 w337 w341 w347 w354 w365 w381 w402 w431 w448 w452 w486 w518 w532 w556 w628 w679 w727 w774 w780] -> w44
      tunnel: w39 -> [w60 w203 w211 w225 w230 w236 w241 w264 w271 w275 w278 w284 w296 w322 w327 w337 w341 w347 w354 w366 w382 w403 w432 w448 w452 w486 w518 w532 w556 w628 w680 w727 w774 w780]
      tunnel: [w63 w204 w209 w227 w233 w238 w242 w266 w272 w276 w280 w286 w297 w323 w328 w338 w342 w348 w355 w376 w384 w405 w441 w449 w453 w455 w505 w533 w557 w629 w689 w728 w777 w781] -> w43
      tunnel: [_ _ _ _ _ TRUE _ _ _ _ _ _ _ _ _ _ _ _ _ _ _ _ _ _ _ _ _ _ _ _ _ _ _ _] -> w38
      tunnel: [w59 w202 w208 w226 w231 w237 w240 w265 w269 w274 w279 w285 w294 w321 w326 w336 w340 w344 w351 w360 w383 w404 w433 w445 w451 w469 w503 w531 w555 w627 w687 w715 w775 w779] -> w42
      tunnel: "update speed [ms]" -> [w58 _ _ _ _ _ _ _ _ _ _ _ _ _ _ _ _ _ _ _ _ _ _ _ _ _ _ _ _ _ _ _ _ _]
      tunnel: w33 -> [w57 _ _ _ _ _ _ _ _ _ _ _ _ _ _ _ _ _ _ _ _ _ _ _ _ _ _ _ _ _ _ _ w772 _]
      tunnel: w32 -> [_ _ _ _ _ _ _ _ _ _ _ _ _ _ _ _ _ _ _ _ _ _ _ _ _ _ _ _ w550 w622 _ _ w776 _]
      frame "", "Idle" {
        # "executes when the state queue is empty"
        n20 = event shown="[2] \"Move Properties\": Value Change" {
          selector: _ -> [_ _ _ _ _ _ _ _ _ _ _ _]
          dyn-events: _ -> [_ _ _ _ _ _ _ _ _ _ _ _]
          timeout: w58 -> [_ _ _ _ _ _ _ _ _ _ _ _]
          tunnel: w64 -> [w90 w128 w133 w140 w148 w153 w157 w162 w169 w179 w195 w201]
          tunnel: [w89 w127 w131 w140 w146 w151 w156 w161 w169 w178 w194 w200] -> w63
          tunnel: w62 -> [w80 w129 w134 w139 w149 w154 w159 w164 w168 w181 w192 w198]
          tunnel: [w86 w126 w130 w141 w145 w150 w158 w163 w170 w182 w193 w199] -> w61
          tunnel: w60 -> [w104 w126 w130 w141 w145 w150 w158 w163 w170 w182 w193 w199]
          tunnel: [w107 w129 w134 w138 w149 w154 w159 w164 w168 w181 w192 w198] -> w59
          tunnel: w57 -> [w66 _ _ _ _ _ _ _ _ _ _ _]
          event Timeout {
            w78 = FALSE ("moving")
            w96 = u32 65421 ("Color")
            n21 = event-data() -> ()  [unwired: 1 in, 1 out]
            n22 = Unbundle By Name(w80) -> ("beam detection para"=w108:T4, "Centriod X"=w106:dbl[], "Centriod Y"=w105:dbl[], "Best Rectangle"=w98:T9)
            n23 = Bundle By Name(cluster=w80, "moving"=w78) -> (w79:T20)
            n24 = local write "moving"(w78) -> ()
            n25 = local read "Target.X::1"() -> (w72:dbl)
            n26 = local read "Target.Y::1"() -> (w71:dbl)
            n27 = call "CENTRIOD DETECTION BEAMPOINTING.vi"("Refnum in"=w66, "beam detection para"=w108, "error in (no error)"=w104) -> ("Bounding Rect"=w74:T21, "Particle Reports (Pixels)"=w83:T8, "Refnum out"=w65:T1, "Centriod"=w75:cluster{"X":dbl, "Y":dbl}, "error out"=w88:errorcluster)  [unwired: 10 in, 2 out]
            "Particle Reports (Pixels)" <- w83
            "Image" <- w65
            n28 = Unbundle By Name(w75) -> ("X"=w101:dbl, "Y"=w100:dbl)
            n29 = Bundle By Name(cluster=T14 {"Draw"=TRUE, "Target"={"x"=25.0, "y"=25.0}, "Size"={"x"=25.0, "y"=25.0}, "Angle"=0.0, "Color"=8322834, "Thickness"=1, "CrosshairLabel"=""} ("Crosshair"), "Target.x"=w72, "Target.y"=w71, "Size"="size 2", "Color"=u32 16774656) -> (w69:T14)
            n30 = Not Equal To 0?(x=w100) -> (x != 0?=w103:bool)
            n31 = Not Equal To 0?(x=w101) -> (x != 0?=w102:bool)
            n32 = Or(x=w102, y=w103) -> (x .or. y?=w99:bool)
            n33 = case shown="True" w99 {
              tunnel: w106 -> [w115 w124]
              tunnel: w105 -> [w114 w123]
              tunnel: [w115 w122] -> w92
              tunnel: [w114 w121] -> w93
              tunnel: w101 -> [_ w120]
              tunnel: w100 -> [_ w119]
              tunnel: w98 -> [w113 w118]
              tunnel: w74 -> [_ w117]
              tunnel: [w113 w116] -> w97
              frame False {
              }
              frame True {
                n34 = Build Array (concatenate)(w118, w117) -> (w116:T9)
                n35 = Build Array (concatenate)(w123, w119) -> (w121:dbl[])
                n36 = Build Array (concatenate)(w124, w120) -> (w122:dbl[])
              }
            }
            "centriod X" <- w92
            "centriod Y" <- w93
            n37 = call "IMAQ Overlay Rectangle"("Color"=w96, "error in (no error)"=w88, "Rectangle"=w74, "Image"=w65) -> ("error out"=w94:errorcluster, "Image Out"=w95:T1)  [unwired: 6 in]
            n38 = call "IMAQ Overlay Points"("Color"=w96, "error in (no error)"=w94, "Point"=w75, "Image"=w95) -> ("error out"=w87:errorcluster, "Image Out"=w67:T1)  [unwired: 6 in]
            n39 = local read "img to avg"() -> (w84:i32)
            n40 = Array Size(array=w92) -> (size(s)=w85:i32)
            n41 = call "draw crosshair imaq.vi"("Crosshair"=w69, "Bounding Rectangle"=T15 {"Left"=0, "Top"=0, "Right"=0, "Bottom"=0}, "image in"=w67) -> ("image out"=→"Beam":T1)  [unwired: 7 in, 1 out]
            n42 = Greater Or Equal?(x=w85, y=w84) -> (x >= y?=w91:bool)
            n43 = case shown="True" w91 {
              tunnel: w90 -> [w109 w112]
              tunnel: [w109 w111] -> w89
              frame False {
              }
              frame True {
                n44 = call <vilib>:"Add State(s) to Queue__jki_lib_state_machine.vi"("State(s) in (\"\")"=w112, "State(s) at Back (\"\")"="detected" ("State(s) in Front (\"\")")) -> ("States Out"=w111:string)  [unwired: 13 in]
              }
            }
            n45 = Empty Array?(array=w83) -> (empty?=w82:bool)
            n46 = Not(x=w82) -> (.not. x?=w81:bool)
            "beam detected" <- w81
            n47 = Bundle By Name(cluster=w79, "PArticle Report"=w83, "Centriod X"=w92, "Centriod Y"=w93, "Best Rectangle"=w97, "beam detected"=w81) -> (w107:T20)
            n48 = call <vilib>:"Clear Errors.vi"("error in (no error)"=w87) -> ("error out"=w86:errorcluster)  [unwired: 5 in, 1 out]
          }
          event Value Change {
            n49 = event-data() -> ()  [unwired: 1 in, 6 out]
            n50 = call <vilib>:"Add State(s) to Queue__jki_lib_state_machine.vi"("State(s) in (\"\")"=w128, "State(s) at Back (\"\")"="Beam Detection" ("State(s) at Back (\"\")")) -> ("States Out"=w127:string)  [unwired: 13 in]
          }
          event Value Change {
            n51 = event-data() -> ()  [unwired: 1 in, 6 out]
            n52 = call <vilib>:"Add State(s) to Queue__jki_lib_state_machine.vi"("State(s) in (\"\")"=w133, "State(s) at Back (\"\")"=" Move Properties" ("State(s) at Back (\"\")")) -> ("States Out"=w131:string)  [unwired: 13 in]
          }
          event "ActiveMotor": Value Change {
            n53 = event-data() -> ("CtlRef"=w143:refnum<vi>, "NewVal"=w142:u16)  [unwired: 1 in, 4 out]
            n54 = property on="Property Node" class="Ring (strict)"(reference=w143) -> ("Strings []"=w144:string[])  [unwired: 1 in, 2 out]
            n55 = local read "Move Properties"() -> (w137:T6)
            n56 = Index Array(array=w144, index=w142) -> (element=w136:string)
            n57 = Bundle By Name(cluster=w137, "my active motor"=w136) -> (w135:T6)
            n58 = Bundle By Name(cluster=w139, "move.my active motor"=w136) -> (w138:T20)
            n59 = local write "Move Properties"(w135) -> ()
            n60 = property on="ActiveMotorName::2" class="Str"("Val(Sgnl)"=w136) -> ()  [unwired: 2 in, 2 out]
          }
          event "Save Config": Value Change {
            n61 = event-data() -> ()  [unwired: 1 in, 6 out]
            n62 = call <vilib>:"Add State(s) to Queue__jki_lib_state_machine.vi"("State(s) in (\"\")"=w148, "State(s) at Back (\"\")"="Save Configuration" ("State(s) in Front (\"\")")) -> ("States Out"=w146:string)  [unwired: 13 in]
          }
          event "Save Stats": Value Change {
            n63 = event-data() -> ()  [unwired: 1 in, 6 out]
            n64 = call <vilib>:"Add State(s) to Queue__jki_lib_state_machine.vi"("State(s) in (\"\")"=w153, "State(s) at Back (\"\")"="Save Stats" ("State(s) in Front (\"\")")) -> ("States Out"=w151:string)  [unwired: 13 in]
          }
          event "Load Config": Value Change {
            n65 = event-data() -> ()  [unwired: 1 in, 6 out]
            n66 = call <vilib>:"Add State(s) to Queue__jki_lib_state_machine.vi"("State(s) in (\"\")"=w157, "State(s) at Back (\"\")"="Load Configuration" ("State(s) in Front (\"\")")) -> ("States Out"=w156:string)  [unwired: 13 in]
          }
          event "Reset History": Value Change {
            n67 = event-data() -> ()  [unwired: 1 in, 6 out]
            n68 = call <vilib>:"Add State(s) to Queue__jki_lib_state_machine.vi"("State(s) in (\"\")"=w162, "State(s) at Back (\"\")"="Reset History" ("State(s) in Front (\"\")")) -> ("States Out"=w161:string)  [unwired: 13 in]
          }
          event "Set Centriod Target": Value Change {
            n69 = event-data() -> ()  [unwired: 1 in, 6 out]
            n70 = Two Button Dialog(message="Do want to update the target?") -> (T button?=w165:bool)  [unwired: 2 in]
            n71 = case shown="True" w165 {
              tunnel: w168 -> [_ w175]
              frame False {
              }
              frame True {
                n72 = Unbundle By Name(w175) -> ("Centriod X"=w174:dbl[], "Centriod Y"=w172:dbl[])
                n73 = Index Array(array=w174) -> (element=w173:dbl)  [unwired: 1 in]
                n74 = Index Array(array=w172) -> (element=w171:dbl)  [unwired: 1 in]
                n75 = property on="Target.Y::1" class="DigNum (strict)"("Val(Sgnl)"=w171) -> ()  [unwired: 2 in, 2 out]
                n76 = property on="Target.X::1" class="DigNum (strict)"("Val(Sgnl)"=w173) -> ()  [unwired: 2 in, 2 out]
              }
            }
            n77 = local write "Set Centriod Target"(FALSE ("Set Centriod Target")) -> ()
          }
          event "calibrate": Value Change {
            n78 = event-data() -> ()  [unwired: 1 in, 6 out]
            n79 = call "Calibration Details"() -> ("Number of Steps"=w177:dbl, "OK"=w176:bool)  [unwired: 17 in, 1 out]
            n80 = local write "calibrate"(FALSE ("Set Centriod Target")) -> ()
            n81 = case shown="True" w176 {
              tunnel: w179 -> [w183 w190]
              tunnel: [w183 w189] -> w178
              tunnel: w177 -> [_ w185]
              frame False {
              }
              frame True {
                n82 = To Word Integer(number=w185) -> (16bit integer=w184:i16)
                n83 = Number To Decimal String(number=w184) -> (decimal integer string=w186:string)  [unwired: 1 in]
                n84 = call <vilib>:"Build State String with Arguments__jki_lib_state_machine.vi"("Arguments (\"\")"=w186, "State"="Calibrate" ("State(s) at Back (\"\")")) -> ("State with Arguments"=w187:string)  [unwired: 4 in]
                n85 = call <vilib>:"Add State(s) to Queue__jki_lib_state_machine.vi"("State(s) in (\"\")"=w190, "State(s) at Back (\"\")"=w187) -> ("States Out"=w189:string)  [unwired: 13 in]
              }
            }
          }
          event "stop": Value Change {
            # "Exit Button Value Change (pressed) Event\n(this executes Macro: Exit to terminate the VI)"
            n86 = event-data() -> ()  [unwired: 1 in, 6 out]
            n87 = call <vilib>:"Add State(s) to Queue__jki_lib_state_machine.vi"("State(s) in Front (\"\")"="Macro: Exit", "State(s) in (\"\")"=w195) -> ("States Out"=w194:string)  [unwired: 13 in]
          }
          event Panel Close? {
            # "Discard the event because we'll close the front panel ourselves in Macro: Exit"
            # "Close Panel button (pressed) Event\n(this executes Macro: Exit to terminate the VI)"
            n88 = event-data() -> ()  [unwired: 1 in, 1 out]
            n89 = call <vilib>:"Add State(s) to Queue__jki_lib_state_machine.vi"("State(s) in Front (\"\")"="Macro: Exit", "State(s) in (\"\")"=w201) -> ("States Out"=w200:string)  [unwired: 13 in]
            n90 = event-data("Discard?"=TRUE) -> ()  [unwired: 1 in, 1 out]
          }
        }
      }
      frame "---------- Core ----------" {
        # "Do not put any code in this frame.\n(it is a separator no-op)"
        n91 = call <vilib>:"Add State(s) to Queue__jki_lib_state_machine.vi"("State(s) in (\"\")"=w205) -> ("States Out"=w204:string)  [unwired: 14 in]
      }
      frame Default {
        w215 = 42 items=["No error", "Argument error", "Memory is full", "Out of zone", "End of file", "File already open", "Generic file I/O error", "File not found", "File permission error", "Disk is full", "Duplicate path", "Too many files open", "System feature not enabled", "Resource file not found", "Cannot add resource", "Resource not found", "Image not found", "Image memory error", "Pen does not exist", "Config type invalid", "Config token not found", "Config parse error", "Config memory error", "Bad external code format", "Bad external code offset", "External code not present", "Null window", "Destroy window error", "Null menu", "Print aborted", "Bad print record", "Print driver error", "Windows error during printing", "Memory error during printing", "Print dialog error", "Generic print error", "Invalid device refnum", "Device not found", "Device parameter error", "Device unit error", "Cannot open device", "Device call aborted", "Generic error", "Cancelled by user", "Object ID too low", "Object ID too high", "Object not in heap", "Unknown heap", "Unknown object (invalid DefProc)", "Unknown object (DefProc not in table)", "Message out of range", "Invalid (null) method", "Unknown message", "Manager call not supported", "Bad address", "Network operation in progress", "Network operation timed out", "Connection is busy", "Network attribute not supported", "Network error", "Address in use", "System out of memory", "Connection aborted", "Connection refused", "Not connected", "Already connected", "Connection closed", "Initialization error (interapplication manager)", "Bad occurrence", "Wait on unbound occurrence handler", "Occurrence queue overflow", "Datalog type conflict", "Unused", "Unrecognized type (interapplication manager)", "Memory corrupt", "Failed to make temporary DLL", "Old CIN version", "Drag socket not found", "Failed to load drop-object", "Failed to register OLE object", "Failed to release OLE object", "Format specifier type mismatch", "Unknown format specifier", "Too few format specifiers", "Too many format specifiers", "Scan failed", "Newer CIN version", "Error converting to variant", "Runtime menu error", "Password tampered", "Variant attribute not found", "Incompatible variant data type", "Event data is not available", "Event Store is not present", "Occurrence is not found", "Event Queue is not created", "Event info is not available", "Refnum passed is NULL", "Error retrieving Class GUID", "Error retrieving CoClass GUID", "Error retrieving TypeLib GUID.", "Bad built application magic bytes.", "Specific driver is different from the specific driver associated with the Logical Name.", "There is no session opened to the class driver.", "Max Error", "MAX - Error with config objects", "MAX - Error loading configuration", "MAX - Group not supported"]
        # "Current State"
        # "Do not delete, rename, or modify this frame.\n(this is used to capture unhandled states and typos)"
        # "Handle mistyped state name (developer tool)"
        n92 = Format Into String(format string="Software Exception: Unhandled State \"%s\"." ("message"), error in=w211, w206) -> (resulting string=w214:string, error out=w213:errorcluster)  [unwired: 1 in]
        n93 = call <vilib>:"Error Cluster From Error Code.vi"("show call chain? (False)"=TRUE, "error in (no error)"=w213, "error message (\"\")"=w214, "error code (0)"=w215) -> ("error out"=w212:errorcluster)  [unwired: 5 in]
        n94 = call <vilib>:"Add State(s) to Queue__jki_lib_state_machine.vi"("State(s) in (\"\")"=w210) -> ("States Out"=w209:string)  [unwired: 14 in]
      }
      frame "Initialize Core Data" {
        # "Do not delete, rename, or modify this frame.\n(this is used to determine panel behavior on exit)"
        # "originally closed?"
        # "exe?"
        # "If panel starts closed or is an EXE, then close it when we exit"
        n95 = property class="VI"() -> ("Front Panel.Open"=w224:bool)  [unwired: 2 in, 2 out]
        n96 = property class="App"() -> ("App.Kind"=w223:T16)  [unwired: 2 in, 2 out]
        n97 = control-ref of="Current VI Reference"() -> (w217:refnum<vi>)
        n98 = Not(x=w224) -> (.not. x?=w221:bool)
        n99 = Equal?(x=w223, y=T16."Run Time System" ("Application:Kind")) -> (x = y?=w220:bool)
        n100 = Or(x=w221, y=w220) -> (x .or. y?=w218:bool)
        n101 = Bundle By Name(cluster=w219, "Core.Current VI Reference"=w217, "Core.Close Panel on Exit?"=w218) -> (w226:T20)
        n102 = call <vilib>:"Add State(s) to Queue__jki_lib_state_machine.vi"("State(s) in (\"\")"=w228) -> ("States Out"=w227:string)  [unwired: 14 in]
      }
      frame "Error Handler" {
        # "Unhandled Error -- Display it"
        # "Handle any errors here.\nYou can also output any states to clean-up after errors occur"
        # "Clear error"
        n103 = call <vilib>:"General Error Handler.vi"("error in (no error)"=w230) -> ()  [unwired: 10 in, 5 out]
        n104 = call <vilib>:"Add State(s) to Queue__jki_lib_state_machine.vi"("State(s) in Front (\"\")"="/* Post Error States", "State(s) in (\"\")"=w234) -> ("States Out"=w233:string)  [unwired: 13 in]
      }
      frame "Exit" {
        # "Do not put any code in this frame.\n(No errors that occur here will be handled.)"
        n105 = call <vilib>:"Add State(s) to Queue__jki_lib_state_machine.vi"("State(s) in (\"\")"=w239) -> ("States Out"=w238:string)  [unwired: 14 in]
      }
      frame "---------- Data ----------" {
        # "Do not put any code in this frame.\n(It is a separator no-op. You can make a copy of this frame to create a new Data frame)"
        n106 = call <vilib>:"Add State(s) to Queue__jki_lib_state_machine.vi"("State(s) in (\"\")"=w243) -> ("States Out"=w242:string)  [unwired: 14 in]
      }
      frame "Data: Initialize" {
        w249 = T19 {"Slope Axis 1"=0.0, "Axis Inverted"=FALSE, "Slope Axis 2"=0.0, "Axis 1 revered"=FALSE, "Axis 2 revered"=FALSE}  # Motor Calibration
        w250 = FALSE  # set centriod target
        w251 = T2 {"Stat Centriod X"=[], "Stat Centriod Y"=[], "TRA Position X"=[], "TRA PositionY"=[], "Time"=[]}  # Stats
        w253 = FALSE  # moving
        w245 = T6 {"Tolerance [%]"=0.0, "Stepsize"=0.0, "Invert Axis"=FALSE, "Invert Direction X"=FALSE, "Invert Direction Y"=FALSE, "enable feedback"=FALSE, "Set Centriod Target"=FALSE, "my active motor"=""}  # move
        w254 = cluster{"X offset":dbl, "Y offset":dbl} {"X offset"=0.0, "Y offset"=0.0}  # offsets
        w255 = FALSE  # beam detected
        w252 = T4 {"Filter"=1, "Filter Para"={"X Size"=5, "Y Size"=5, "% Tolerance"=1}, "detection method"=4, "smal para"=[{"Measurement Parameter"=35, "Range Lower Value"=0.0, "Range Upper Value"=500.0, "Range"=TRUE, "Measurement Type"=FALSE}], "Remove small Objects"=TRUE, "Restrict to round Objects"=FALSE}  # beam detection para
        w257 = dbl[] []  # Mean Centriod Y
        w258 = dbl[] []  # Mean Centriod X
        w259 = T8 [{"Area"=1104.0, "Number of Holes"=0.0, "Bounding Rect"={"Left"=378.0, "Top"=230.0, "Right"=422.0, "Bottom"=264.0}, "Center of Mass"={"X"=399.60235507246375, "Y"=246.169384057971}, "Orientation"=6.346766143267859, "Dimensions"={"Width"=44.0, "Height"=34.0}}]  # PArticle Report
        w260 = T9 []  # Best Rectangle
        w261 = dbl[] []  # Centriod Y
        w262 = dbl[] []  # Centriod X
        w263 = T22 {"Current VI Reference"=refnum, "Close Panel on Exit?"=FALSE}  # Core
        # "Initialize the shift-register data, here.\n(data names are defined by what you wire into the bundle function)"
        n107 = local read "ActiveMotor"() -> (w247:u16)
        n108 = local write "beam detection para"(w252) -> ()
        n109 = property on="ActiveMotor" class="Ring (strict)"() -> ("Strings []"=w248:string[])  [unwired: 2 in, 2 out]
        n110 = Bundle("Core"=w263, "beam detection para"=w252, "Centriod X"=w262, "Centriod Y"=w261, "Best Rectangle"=w260, "PArticle Report"=w259, "Mean Centriod X"=w258, "Mean Centriod Y"=w257, "Time"="Time", "beam detected"=w255, "offsets"=w254, "move"=w245, "moving"=w253, "Stats"=w251, "set centriod target"=w250, "Motor Calibration"=w249) -> (w265:T20)  [unwired: 1 in]
        n111 = Index Array(array=w248, index=w247) -> (element=w246:string)
        n112 = Bundle By Name(cluster=w245, "my active motor"=w246) -> (w244:T6)
        n113 = property on="ActiveMotorName::2" class="Str"("Val(Sgnl)"=w246) -> ()  [unwired: 2 in, 2 out]
        n114 = call <vilib>:"Add State(s) to Queue__jki_lib_state_machine.vi"("State(s) in (\"\")"=w267) -> ("States Out"=w266:string)  [unwired: 14 in]
        n115 = property on="Move Properties" class="Clust (strict)"("Value"=w244) -> ()  [unwired: 2 in, 2 out]
      }
      frame "Data: Cleanup" {
        # "Cleanup any data and references, here.\n(this is called automatically, by the Macro: Exit)"
        n116 = Unbundle By Name(w269) -> ("Core.Current VI Reference"=w268:refnum<vi>)
        n117 = Close Reference(reference=w268, error in (no error)=w271) -> (error out=w270:errorcluster)
        n118 = call <vilib>:"Add State(s) to Queue__jki_lib_state_machine.vi"("State(s) in (\"\")"=w273) -> ("States Out"=w272:string)  [unwired: 14 in]
      }
      frame "---------- UI ----------" {
        # "Do not put any code in this frame.\n(It is a separator no-op. You can make a copy of this frame to create a new UI frame)"
        n119 = call <vilib>:"Add State(s) to Queue__jki_lib_state_machine.vi"("State(s) in (\"\")"=w277) -> ("States Out"=w276:string)  [unwired: 14 in]
      }
      frame "UI: Initialize" {
        # "Initialize the User Interface, here.\n(this is called automatically, by the Macro: Init)"
        n120 = call <vilib>:"Add State(s) to Queue__jki_lib_state_machine.vi"("State(s) in (\"\")"=w281) -> ("States Out"=w280:string)  [unwired: 14 in]
      }
      frame "UI: Cursor Set" {
        # "Argument"
        # "Set and Unset Cursor Busy.\n(Usage: \"UI: Cursor Set >> Busy|Idle\")"
        n121 = case shown="\"Idle\", Default" w282 {
          tunnel: w284 -> [w289 w291]
          tunnel: [w288 w290] -> w283
          frame "Idle", Default {
            n122 = call <vilib>:"Unset Busy.vi"("error in (no error)"=w289) -> ("error out"=w288:errorcluster)  [unwired: 10 in]
          }
          frame "Busy" {
            n123 = call <vilib>:"Set Busy.vi"("error in (no error)"=w291) -> ("error out"=w290:errorcluster)  [unwired: 9 in, 1 out]
          }
        }
        n124 = call <vilib>:"Add State(s) to Queue__jki_lib_state_machine.vi"("State(s) in (\"\")"=w287) -> ("States Out"=w286:string)  [unwired: 14 in]
      }
      frame "UI: Front Panel State" {
        # "Argument"
        # "Set Front Panel Open or Closed\n(Usage: \"UI: Front Panel State >> Open|Close\")"
        n125 = Unbundle By Name(w294) -> ("Core.Current VI Reference"=w293:refnum<vi>)
        n126 = case shown="\"Close\"" w292 {
          tunnel: w296 -> [w302 w315]
          tunnel: [w304 w316] -> w295
          tunnel: w293 -> [w303 w313]
          frame "Open", Default {
            n127 = property class="VI"(reference=w303, error in=w302) -> (reference out=w300:refnum<vi>, error out=w301:errorcluster, "Front Panel.Open"=w299:bool)
            n128 = case shown="False" w299 {
              tunnel: [w307 w310] -> w304
              tunnel: w301 -> [w306 w310]
              tunnel: w300 -> [w305 _]
              frame False {
                n129 = invoke class="VI" method="FP.Open"(reference=w305, error in=w306, "Activate"=TRUE, "State"=T17."Standard") -> (error out=w307:errorcluster)  [unwired: 1 in, 4 out]
              }
              frame True {
              }
            }
          }
          frame "Close" {
            n130 = property class="VI"(reference=w313, error in=w315) -> (reference out=w312:refnum<vi>, error out=w314:errorcluster, "Front Panel.Open"=w311:bool)
            n131 = case shown="True" w311 {
              tunnel: [w317 w320] -> w316
              tunnel: w314 -> [w317 w319]
              tunnel: w312 -> [_ w318]
              frame False {
              }
              frame True {
                n132 = invoke class="VI" method="FP.Close"(reference=w318, error in=w319) -> (error out=w320:errorcluster)  [unwired: 1 in, 2 out]
              }
            }
          }
        }
        n133 = call <vilib>:"Add State(s) to Queue__jki_lib_state_machine.vi"("State(s) in (\"\")"=w298) -> ("States Out"=w297:string)  [unwired: 14 in]
      }
      frame "---------- Macro ----------" {
        # "Do not put any code in this frame.\n(It is a separator no-op. You can make a copy of this frame to create a new Macro frame)"
        n134 = call <vilib>:"Add State(s) to Queue__jki_lib_state_machine.vi"("State(s) in (\"\")"=w324) -> ("States Out"=w323:string)  [unwired: 14 in]
      }
      frame "Macro: Initialize" {
        w325 = "Data: Initialize\nInitialize Core Data\nUI: Initialize\nUI: Front Panel State >> Open"  # Data: Initialize Initialize Core Data UI: Initialize UI: Front Panel State >> Open
        # "Initialization Macro\n(This is called once, when the VI starts)"
        n135 = call <vilib>:"Add State(s) to Queue__jki_lib_state_machine.vi"("State(s) in Front (\"\")"=w325, "State(s) in (\"\")"=w329) -> ("States Out"=w328:string)  [unwired: 13 in]
      }
      frame "Macro: Exit" {
        # "Exit Macro\n(This is called once, when the VI exits)"
        n136 = Unbundle By Name(w336) -> ("Core.Close Panel on Exit?"=w334:bool)
        n137 = Select(t="UI: Front Panel State >> Close", s=w334, f="") -> (s? t:f=w331:string)
        n138 = call <vilib>:"Add State(s) to Queue__jki_lib_state_machine.vi"("State(s) in (\"\")"=w331, "State(s) at Back (\"\")"="Data: Cleanup\nExit") -> ("States Out"=w335:string)  [unwired: 13 in]
        n139 = call <vilib>:"Add State(s) to Queue__jki_lib_state_machine.vi"("State(s) in Front (\"\")"=w335, "State(s) in (\"\")"=w339) -> ("States Out"=w338:string)  [unwired: 13 in]
      }
      frame "-------------Properties---------" {
        # "Template Separator\n(You can make a copy of, or modify, this frame)"
        n140 = call <vilib>:"Add State(s) to Queue__jki_lib_state_machine.vi"("State(s) in (\"\")"=w343) -> ("States Out"=w342:string)  [unwired: 14 in]
      }
      frame "Beam Detection" {
        # "Your code here.\n(You can make a copy of, or modify, this frame)"
        n141 = Bundle By Name(cluster=w345, "beam detection para"="beam detection para") -> (w344:T20)
        n142 = call <vilib>:"Add State(s) to Queue__jki_lib_state_machine.vi"("State(s) in (\"\")"=w349) -> ("States Out"=w348:string)  [unwired: 14 in]
      }
      frame "Move Properties" {
        n143 = Bundle By Name(cluster=w352, "move"="Move Properties") -> (w351:T20)
        n144 = Unbundle By Name(w351) -> ("move.Stepsize"=w350:dbl)
        n145 = property on="RelativeSettings.Axis 1.StepSize::2" class="DigNum (strict)"("Val(Sgnl)"=w350) -> ()  [unwired: 2 in, 2 out]
        n146 = property on="RelativeSettings.Axis 2.StepSize::2" class="DigNum (strict)"("Val(Sgnl)"=w350) -> ()  [unwired: 2 in, 2 out]
        n147 = call <vilib>:"Add State(s) to Queue__jki_lib_state_machine.vi"("State(s) in (\"\")"=w356) -> ("States Out"=w355:string)  [unwired: 14 in]
      }
      frame "Save Configuration" {
        n148 = Bundle By Name(cluster=w360, "move.enable feedback"=FALSE) -> (w358:T20)
        n149 = local read "GUIdevice 1"() -> (w363:string)
        n150 = local read "ActiveMotor"() -> (w361:u16)
        n151 = local read "GUIdevice 2"() -> (w362:string)
        n152 = local read "stats path"() -> (w357:path)
        n153 = Unbundle By Name(w358) -> ("beam detection para"=w372:T4, "move"=w371:T6)
        n154 = local read "img to avg"() -> (w373:i32)
        n155 = Bundle("img to avg"=w373, "beam detection para"=w372, "move"=w371, "GUIdevice 1"=w363, "GUIdevice 2"=w362, "ActiveMotor"=w361, "stats path"=w357) -> (w370:T7)  [unwired: 1 in]
        n156 = Open/Create/Replace File(error in=w366, operation (0:open)=T18."replace or create with confirmation") -> (refnum out=w374:refnum<file>, error out=w369:errorcluster)  [unwired: 4 in, 1 out]
        n157 = Write to Binary File(file (use dialog)=w374, data=w370, error in=w369) -> (refnum out=w367:refnum<file>, error out=w368:errorcluster)  [unwired: 3 in, 1 out]
        n158 = Close File(refnum=w367, error in=w368) -> (error out=w365:errorcluster)  [unwired: 1 out]
        n159 = local write "Save Config"(FALSE ("Save Button")) -> ()
        n160 = call <vilib>:"Add State(s) to Queue__jki_lib_state_machine.vi"("State(s) in (\"\")"=w377) -> ("States Out"=w376:string)  [unwired: 14 in]
      }
      frame "Save Stats" {
        n161 = local read "Save Stats"() -> (w378:bool)
        n162 = Unbundle By Name(w383) -> ("Stats"=w379:T2)
        n163 = case shown="True" w378 {
          tunnel: w382 -> [w386 w390]
          tunnel: [w386 w389] -> w381
          tunnel: w379 -> [_ w388]
          frame False {
          }
          frame True {
            n164 = Open/Create/Replace File(file path (use dialog)="stats path", error in=w390, operation (0:open)=T18."replace or create") -> (refnum out=w394:refnum<file>, error out=w393:errorcluster)  [unwired: 3 in, 1 out]
            n165 = Write to Binary File(file (use dialog)=w394, data=w388, error in=w393) -> (refnum out=w391:refnum<file>, error out=w392:errorcluster)  [unwired: 3 in, 1 out]
            n166 = Close File(refnum=w391, error in=w392) -> (error out=w389:errorcluster)  [unwired: 1 out]
          }
        }
        n167 = call <vilib>:"Add State(s) to Queue__jki_lib_state_machine.vi"("State(s) in (\"\")"=w385) -> ("States Out"=w384:string)  [unwired: 14 in]
        n168 = local write "Save Stats"(FALSE ("Save Button")) -> ()
      }
      frame "Save Centriod" {
        n169 = local read "Save Stats"() -> (w396:bool)
        n170 = Unbundle By Name(w404) -> ("Time"=w400:timestamp[], "Mean Centriod X"=w399:dbl[], "Mean Centriod Y"=w398:dbl[])
        n171 = Bundle("Time"=w400, "Mean Centriod X"=w399, "Mean Centriod Y"=w398) -> (w397:T3)  [unwired: 1 in]
        n172 = case shown="True" w396 {
          tunnel: w403 -> [w407 w416]
          tunnel: [w407 w415] -> w402
          tunnel: w397 -> [_ w408]
          frame False {
          }
          frame True {
            n173 = local read "stats path"() -> (w414:path)
            n174 = Strip Path(path=w414) -> (stripped path=w410:path, name=w413:string)
            n175 = Concatenate Strings("Centriod_" ("string"), w413) -> (w411:string)
            n176 = Build Path(base path=w410, name or relative path=w411) -> (appended path=w409:path)
            n177 = Open/Create/Replace File(file path (use dialog)=w409, error in=w416, operation (0:open)=T18."replace or create") -> (refnum out=w420:refnum<file>, error out=w419:errorcluster)  [unwired: 3 in, 1 out]
            n178 = Write to Binary File(file (use dialog)=w420, data=w408, error in=w419) -> (refnum out=w417:refnum<file>, error out=w418:errorcluster)  [unwired: 3 in, 1 out]
            n179 = Close File(refnum=w417, error in=w418) -> (error out=w415:errorcluster)  [unwired: 1 out]
          }
        }
        n180 = call <vilib>:"Add State(s) to Queue__jki_lib_state_machine.vi"("State(s) in (\"\")"=w406) -> ("States Out"=w405:string)  [unwired: 14 in]
        n181 = local write "Save Stats"(FALSE ("Save Button")) -> ()
      }
      frame "Load Configuration" {
        # "Your code here.\n(You can make a copy of, or modify, this frame)"
        n182 = Open/Create/Replace File(error in=w432, operation (0:open)=T18."open") -> (refnum out=w439:refnum<file>, error out=w438:errorcluster)  [unwired: 4 in, 1 out]
        n183 = Read from Binary File(5:"output cluster", 8:w438, 11:w439) -> (0:w437:errorcluster, 2:w435:T7, 3:w436:refnum<file>)  [unwired: 3 in, 1 out]
        n184 = Close File(refnum=w436, error in=w437) -> (error out=w431:errorcluster)  [unwired: 1 out]
        n185 = Unbundle By Name(w435) -> ("img to avg"=w424:i32, "beam detection para"=w430:T4, "move"=w429:T6, "GUIdevice 1"=w427:string, "GUIdevice 2"=w426:string, "ActiveMotor"=w423:u16, "stats path"=w422:path)
        n186 = local write "img to avg"(w424) -> ()
        n187 = property on="GUIdevice 2" class="Str"("Val(Sgnl)"=w426) -> ()  [unwired: 2 in, 2 out]
        n188 = local write "ActiveMotor"(w423) -> ()
        n189 = local write "stats path"(w422) -> ()
        n190 = property on="GUIdevice 1" class="Str"("Val(Sgnl)"=w427) -> ()  [unwired: 2 in, 2 out]
        n191 = call <vilib>:"Add State(s) to Queue__jki_lib_state_machine.vi"("State(s) in (\"\")"=w442) -> ("States Out"=w441:string)  [unwired: 14 in]
        n192 = Bundle By Name(cluster=w434, "beam detection para"=w430, "move"=w429) -> (w433:T20)
        n193 = local write "Load Config"(FALSE ("Load Button")) -> ()
        n194 = local write "beam detection para"(w430) -> ()
        n195 = local write "Move Properties"(w429) -> ()
      }
      frame "Reset History" {
        w447 = dbl[] [] ("Mean Centriod X")
        # "Your code here.\n(You can make a copy of, or modify, this frame)"
        n196 = local write "Reset History"(FALSE ("Reset History")) -> ()
        n197 = call <vilib>:"Add State(s) to Queue__jki_lib_state_machine.vi"("State(s) in (\"\")"=w450) -> ("States Out"=w449:string)  [unwired: 14 in]
        n198 = Bundle By Name(cluster=w446, "Mean Centriod X"=w447, "Mean Centriod Y"=w447, "Stats"=T2 {"Stat Centriod X"=[], "Stat Centriod Y"=[], "TRA Position X"=[], "TRA PositionY"=[], "Time"=[]}) -> (w445:T20)
      }
      frame "---------- centriod analysis----------" {
        # "Template Separator\n(You can make a copy of, or modify, this frame)"
        n199 = call <vilib>:"Add State(s) to Queue__jki_lib_state_machine.vi"("State(s) in (\"\")"=w454) -> ("States Out"=w453:string)  [unwired: 14 in]
      }
      frame "detected" {
        w460 = 101 ("y")
        w485 = dbl[] [] ("Array")
        n200 = Unbundle By Name(w470) -> ("Time"=w478:timestamp[], "Centriod X"=w473:dbl[], "Mean Centriod X"=w477:dbl[], "Centriod Y"=w472:dbl[], "Mean Centriod Y"=w476:dbl[], "Best Rectangle"=→"Best Rectangle":T9)
        n201 = local read "Target.X::1"() -> (w475:dbl)
        n202 = local read "Target.Y::1"() -> (w474:dbl)
        n203 = call <vilib>:"Std Deviation and Variance.vi"("X"=w473) -> ("mean"=w479:dbl)  [unwired: 1 in, 2 out]
        "mean X" <- w479
        n204 = call <vilib>:"Std Deviation and Variance.vi"("X"=w472) -> ("mean"=w480:dbl)  [unwired: 1 in, 2 out]
        "mean Y" <- w480
        n205 = Subtract(x=w475, y=w479) -> (x-y=w468:dbl)
        "X offset" <- w468
        n206 = Subtract(x=w474, y=w480) -> (x-y=w467:dbl)
        "Y offset" <- w467
        n207 = Get Date/Time In Seconds() -> (seconds since 1Jan1904=w481:timestamp)
        n208 = Build Array (concatenate)(w477, w468) -> (w457:dbl[])
        n209 = Build Array (concatenate)(w476, w467) -> (w458:dbl[])
        n210 = Build Array (concatenate)(w478, w481) -> (w471:timestamp[])
        n211 = Bundle(w468, w467) -> (w466:cluster{dbl, dbl})  [unwired: 1 in]
        n212 = Array Size(array=w457) -> (size(s)=w462:i32)
        n213 = call <vilib>:"Add State(s) to Queue__jki_lib_state_machine.vi"("State(s) in (\"\")"=w487, "State(s) at Back (\"\")"="check move") -> ("States Out"=w456:string)  [unwired: 13 in]
        n214 = Decrement(x=w460) -> (x-1=w459:i32)
        n215 = Quotient & Remainder(x=w462, y=w460) -> (x-y*floor(x/y)=w461:i32)  [unwired: 1 out]
        n216 = Bundle(w471, w457) -> (w482:cluster{timestamp[], dbl[]})  [unwired: 1 in]
        n217 = Bundle(w471, w458) -> (w483:cluster{timestamp[], dbl[]})  [unwired: 1 in]
        n218 = Equal?(x=w461, y=w459) -> (x = y?=w463:bool)
        n219 = Build Array(w482, w483) -> (→"XY Graph":cluster{timestamp[], dbl[]}[])
        n220 = case shown="True" w463 {
          tunnel: [w488 w490] -> w455
          tunnel: w456 -> [w488 w489]
          frame False {
          }
          frame True {
            n221 = call <vilib>:"Add State(s) to Queue__jki_lib_state_machine.vi"("State(s) in Front (\"\")"=w489, "State(s) at Back (\"\")"="Save Centriod" ("State(s) at Back (\"\")")) -> ("States Out"=w490:string)  [unwired: 13 in]
          }
        }
        n222 = Bundle By Name(cluster=w470, "Time"=w471, "Mean Centriod X"=w457, "Mean Centriod Y"=w458, "Centriod X"=w485, "Centriod Y"=w485, "offsets"=w466) -> (w469:T20)
      }
      frame "check move" {
        n223 = Unbundle By Name(w499) -> ("Best Rectangle"=w517:T9, "offsets.X offset"=w516:dbl, "offsets.Y offset"=w515:dbl)
        n224 = Absolute Value(x=w516) -> (abs(x)=w512:dbl)
        n225 = Absolute Value(x=w515) -> (abs(x)=w509:dbl)
        n226 = Unbundle By Name(w499) -> ("move.Tolerance [%]"=w514:dbl)
        n227 = call "Beam Size.vi"("Best Rectangle"=w517) -> ("Y Size"=w495:dbl, "X Size"=w496:dbl)  [unwired: 9 in]
        "X Size" <- w496
        "Y Size" <- w495
        n228 = Divide(x=w514, y=100.0) -> (x/y=w510:dbl)
        n229 = Max & Min(x=w496, y=w495) -> (max(x,y)=w494:dbl)  [unwired: 1 out]
        n230 = Multiply(x=w510, y=w496) -> (x*y=w511:dbl)
        n231 = Multiply(x=w510, y=w495) -> (x*y=w508:dbl)
        n232 = Divide(x=w494, y=2.0) -> (x/y=w492:dbl)
        n233 = local write "size"(w492) -> ()
        n234 = Greater Or Equal?(x=w512, y=w511) -> (x >= y?=w502:bool)
        n235 = Greater Or Equal?(x=w509, y=w508) -> (x >= y?=w501:bool)
        n236 = Unbundle By Name(w499) -> ("move.enable feedback"=w498:bool)
        n237 = case shown="True" w501 {
          tunnel: w497 -> [w523 w526]
          tunnel: [w523 w524] -> w507
          frame False {
          }
          frame True {
            n238 = call <vilib>:"Add State(s) to Queue__jki_lib_state_machine.vi"("State(s) in (\"\")"=w526, "State(s) at Back (\"\")"="Move Y" ("State(s) at Back (\"\")")) -> ("States Out"=w524:string)  [unwired: 13 in]
          }
        }
        n239 = case shown="True" w502 {
          tunnel: w497 -> [w527 w530]
          tunnel: [w527 w528] -> w506
          frame False {
          }
          frame True {
            n240 = call <vilib>:"Add State(s) to Queue__jki_lib_state_machine.vi"("State(s) in (\"\")"=w530, "State(s) at Back (\"\")"="Move X" ("State(s) at Back (\"\")")) -> ("States Out"=w528:string)  [unwired: 13 in]
          }
        }
        n241 = Or(x=w502, y=w501) -> (x .or. y?=w500:bool)
        n242 = local write "move required"(w500) -> ()
        n243 = Bundle By Name(cluster=w499, "Best Rectangle"=T9 []) -> (w503:T20)
        n244 = case shown="True" w498 {
          tunnel: w507 -> [_ w522]
          tunnel: w506 -> [_ w521]
          tunnel: [w519 w520] -> w505
          tunnel: w497 -> [w519 _]
          frame False {
          }
          frame True {
            n245 = call <vilib>:"Add State(s) to Queue__jki_lib_state_machine.vi"("State(s) in (\"\")"=w521, "State(s) at Back (\"\")"=w522) -> ("States Out"=w520:string)  [unwired: 13 in]
          }
        }
      }
      frame "-----------Motor Move---------" {
        # "Your code here.\n(You can make a copy of, or modify, this frame)"
        n246 = call <vilib>:"Add State(s) to Queue__jki_lib_state_machine.vi"("State(s) in (\"\")"=w534) -> ("States Out"=w533:string)  [unwired: 14 in]
      }
      frame "Move X" {
        w554 = TRUE ("moving")
        n247 = Unbundle By Name(w550) -> ("RelativeMove.Axis 1.CW::2"=w549:refnum<vi>, "RelativeMove.Axis 1.CCW::2"=w548:refnum<vi>, "RelativeMove.Axis 2.CW::2"=w547:refnum<vi>, "RelativeMove.Axis 2.CCW::2"=w546:refnum<vi>)
        n248 = Unbundle By Name(w545) -> ("move.Invert Direction X"=w551:bool, "move.Invert Axis"=w552:bool, "offsets.X offset"=w553:dbl)
        n249 = Greater Than 0?(x=w553) -> (x > 0?=w543:bool)
        n250 = Unbundle By Name(w545) -> ("move.my active motor"=w544:string)
        n251 = stacked-sequence {
          tunnel: w543 -> [_ w566]
          tunnel: w552 -> [_ w565]
          tunnel: w551 -> [_ w564]
          tunnel: w549 -> [_ w563]
          tunnel: w548 -> [_ w562]
          tunnel: w547 -> [_ w561]
          tunnel: w546 -> [_ w560]
          tunnel: w544 -> [w559 _]
          frame #0 {
            n252 = property on="ActiveMotorName::2" class="Str"("Val(Sgnl)"=w559) -> ()  [unwired: 2 in, 2 out]
          }
          frame #1 {
            n253 = case shown="False" w566 {
              tunnel: w565 -> [w572 w592]
              tunnel: w564 -> [w571 w591]
              tunnel: w563 -> [w570 w589]
              tunnel: w562 -> [w569 w590]
              tunnel: w561 -> [w568 w588]
              tunnel: w560 -> [w567 w587]
              frame True {
                n254 = case shown="False" w572 {
                  tunnel: w571 -> [w575 w582]
                  tunnel: w570 -> [w574 _]
                  tunnel: w569 -> [w573 _]
                  tunnel: w568 -> [_ w581]
                  tunnel: w567 -> [_ w580]
                  frame False {
                    n255 = case shown="False" w575 {
                      tunnel: w574 -> [w577 _]
                      tunnel: w573 -> [_ w578]
                      frame False {
                        n256 = property class="Bool (strict)"(reference=w577, "Val(Sgnl)"=TRUE ("Value (Signaling)")) -> ()  [unwired: 1 in, 2 out]
                      }
                      frame True {
                        n257 = property class="Bool (strict)"(reference=w578, "Val(Sgnl)"=TRUE ("Value (Signaling)")) -> ()  [unwired: 1 in, 2 out]
                      }
                    }
                  }
                  frame True {
                    n258 = case shown="False" w582 {
                      tunnel: w581 -> [w583 _]
                      tunnel: w580 -> [_ w585]
                      frame False {
                        n259 = property class="Bool (strict)"(reference=w583, "Val(Sgnl)"=TRUE ("Value (Signaling)")) -> ()  [unwired: 1 in, 2 out]
                      }
                      frame True {
                        n260 = property class="Bool (strict)"(reference=w585, "Val(Sgnl)"=TRUE ("Value (Signaling)")) -> ()  [unwired: 1 in, 2 out]
                      }
                    }
                  }
                }
              }
              frame False {
                n261 = case shown="False" w592 {
                  tunnel: w591 -> [w595 w602]
                  tunnel: w590 -> [w594 _]
                  tunnel: w589 -> [w593 _]
                  tunnel: w588 -> [_ w601]
                  tunnel: w587 -> [_ w600]
                  frame False {
                    n262 = case shown="False" w595 {
                      tunnel: w594 -> [w596 _]
                      tunnel: w593 -> [_ w598]
                      frame False {
                        n263 = property class="Bool (strict)"(reference=w596, "Val(Sgnl)"=TRUE ("Value (Signaling)")) -> ()  [unwired: 1 in, 2 out]
                      }
                      frame True {
                        n264 = property class="Bool (strict)"(reference=w598, "Val(Sgnl)"=TRUE ("Value (Signaling)")) -> ()  [unwired: 1 in, 2 out]
                      }
                    }
                  }
                  frame True {
                    n265 = case shown="True" w602 {
                      tunnel: w601 -> [w603 _]
                      tunnel: w600 -> [_ w605]
                      frame False {
                        n266 = property class="Bool (strict)"(reference=w603, "Val(Sgnl)"=TRUE ("Value (Signaling)")) -> ()  [unwired: 1 in, 2 out]
                      }
                      frame True {
                        n267 = property class="Bool (strict)"(reference=w605, "Val(Sgnl)"=TRUE ("Value (Signaling)")) -> ()  [unwired: 1 in, 2 out]
                      }
                    }
                  }
                }
              }
            }
          }
        }
        n268 = Select(t="pos", s=w543, f="neg") -> (s? t:f=w540:string)
        n269 = Concatenate Strings("x" ("string"), w540) -> (w538:string)
        n270 = call <vilib>:"Build State String with Arguments__jki_lib_state_machine.vi"("Arguments (\"\")"=w538, "State"="Stats") -> ("State with Arguments"=w536:string)  [unwired: 4 in]
        n271 = call <vilib>:"Add State(s) to Queue__jki_lib_state_machine.vi"("State(s) in Front (\"\")"="Wait", "State(s) in (\"\")"=w558, "State(s) at Back (\"\")"=w536) -> ("States Out"=w557:string)  [unwired: 12 in]
        n272 = Bundle By Name(cluster=w545, "moving"=w554) -> (w555:T20)
        n273 = local write "moving"(w554) -> ()
      }
      frame "Move Y" {
        w626 = TRUE ("moving")
        n274 = Unbundle By Name(w622) -> ("RelativeMove.Axis 2.CW::2"=w621:refnum<vi>, "RelativeMove.Axis 2.CCW::2"=w620:refnum<vi>, "RelativeMove.Axis 1.CW::2"=w619:refnum<vi>, "RelativeMove.Axis 1.CCW::2"=w618:refnum<vi>)
        n275 = Unbundle By Name(w617) -> ("move.Invert Direction Y"=w623:bool, "move.Invert Axis"=w624:bool, "offsets.Y offset"=w625:dbl)
        n276 = Greater Than 0?(x=w625) -> (x > 0?=w611:bool)
        n277 = Unbundle By Name(w617) -> ("move.my active motor"=w616:string)
        n278 = stacked-sequence {
          tunnel: w611 -> [_ w638]
          tunnel: w624 -> [_ w637]
          tunnel: w623 -> [_ w636]
          tunnel: w621 -> [_ w635]
          tunnel: w620 -> [_ w634]
          tunnel: w619 -> [_ w633]
          tunnel: w618 -> [_ w632]
          tunnel: w616 -> [w631 _]
          frame #0 {
            n279 = property on="ActiveMotorName::2" class="Str"("Val(Sgnl)"=w631) -> ()  [unwired: 2 in, 2 out]
          }
          frame #1 {
            n280 = case shown="False" w638 {
              tunnel: w637 -> [w644 w664]
              tunnel: w636 -> [w643 w663]
              tunnel: w635 -> [w642 w661]
              tunnel: w634 -> [w641 w662]
              tunnel: w633 -> [w640 w660]
              tunnel: w632 -> [w639 w659]
              frame True {
                n281 = case shown="True" w644 {
                  tunnel: w643 -> [w647 w654]
                  tunnel: w642 -> [w646 _]
                  tunnel: w641 -> [w645 _]
                  tunnel: w640 -> [_ w653]
                  tunnel: w639 -> [_ w652]
                  frame False {
                    n282 = case shown="False" w647 {
                      tunnel: w646 -> [w649 _]
                      tunnel: w645 -> [_ w650]
                      frame False {
                        n283 = property class="Bool (strict)"(reference=w649, "Val(Sgnl)"=TRUE ("Value (Signaling)")) -> ()  [unwired: 1 in, 2 out]
                      }
                      frame True {
                        n284 = property class="Bool (strict)"(reference=w650, "Val(Sgnl)"=TRUE ("Value (Signaling)")) -> ()  [unwired: 1 in, 2 out]
                      }
                    }
                  }
                  frame True {
                    n285 = case shown="True" w654 {
                      tunnel: w653 -> [w655 _]
                      tunnel: w652 -> [_ w657]
                      frame False {
                        n286 = property class="Bool (strict)"(reference=w655, "Val(Sgnl)"=TRUE ("Value (Signaling)")) -> ()  [unwired: 1 in, 2 out]
                      }
                      frame True {
                        n287 = property class="Bool (strict)"(reference=w657, "Val(Sgnl)"=TRUE ("Value (Signaling)")) -> ()  [unwired: 1 in, 2 out]
                      }
                    }
                  }
                }
              }
              frame False {
                n288 = case shown="False" w664 {
                  tunnel: w663 -> [w667 w674]
                  tunnel: w662 -> [w666 _]
                  tunnel: w661 -> [w665 _]
                  tunnel: w660 -> [_ w673]
                  tunnel: w659 -> [_ w672]
                  frame False {
                    n289 = case shown="False" w667 {
                      tunnel: w666 -> [w668 _]
                      tunnel: w665 -> [_ w670]
                      frame False {
                        n290 = property class="Bool (strict)"(reference=w668, "Val(Sgnl)"=TRUE ("Value (Signaling)")) -> ()  [unwired: 1 in, 2 out]
                      }
                      frame True {
                        n291 = property class="Bool (strict)"(reference=w670, "Val(Sgnl)"=TRUE ("Value (Signaling)")) -> ()  [unwired: 1 in, 2 out]
                      }
                    }
                  }
                  frame True {
                    n292 = case shown="True" w674 {
                      tunnel: w673 -> [w675 _]
                      tunnel: w672 -> [_ w677]
                      frame False {
                        n293 = property class="Bool (strict)"(reference=w675, "Val(Sgnl)"=TRUE ("Value (Signaling)")) -> ()  [unwired: 1 in, 2 out]
                      }
                      frame True {
                        n294 = property class="Bool (strict)"(reference=w677, "Val(Sgnl)"=TRUE ("Value (Signaling)")) -> ()  [unwired: 1 in, 2 out]
                      }
                    }
                  }
                }
              }
            }
          }
        }
        n295 = Select(t="pos", s=w611, f="neg") -> (s? t:f=w613:string)
        n296 = Concatenate Strings("y" ("string"), w613) -> (w609:string)
        n297 = call <vilib>:"Build State String with Arguments__jki_lib_state_machine.vi"("Arguments (\"\")"=w609, "State"="Stats") -> ("State with Arguments"=w607:string)  [unwired: 4 in]
        n298 = call <vilib>:"Add State(s) to Queue__jki_lib_state_machine.vi"("State(s) in Front (\"\")"="Wait", "State(s) in (\"\")"=w630, "State(s) at Back (\"\")"=w607) -> ("States Out"=w629:string)  [unwired: 12 in]
        n299 = Bundle By Name(cluster=w617, "moving"=w626) -> (w627:T20)
        n300 = local write "moving"(w626) -> ()
      }
      frame "Wait" {
        w688 = TRUE ("moving")
        # "Wait as long as the motor is moving"
        n301 = Unbundle By Name(w686) -> ("move.Stepsize"=w685:dbl)
        n302 = Multiply(x=w685, y=1.0) -> (x*y=w683:dbl)
        n303 = Add(x=w683, y=100.0) -> (x+y=w681:dbl)
        n304 = call <userlib>:"Wait (ms)__ogtk.vi"("error in (no error)"=w680, "milliseconds to wait"=w681) -> ("error out"=w679:errorcluster)  [unwired: 8 in, 1 out]
        n305 = call <vilib>:"Add State(s) to Queue__jki_lib_state_machine.vi"("State(s) in (\"\")"=w690) -> ("States Out"=w689:string)  [unwired: 14 in]
        n306 = Bundle By Name(cluster=w686, "moving"=w688) -> (w687:T20)
        n307 = local write "moving"(w688) -> ()
      }
      frame "Stats" {
        w698 = 21 ("y")
        # "Your code here.\n(You can make a copy of, or modify, this frame)"
        n308 = Unbundle By Name(w725) -> ("move.Stepsize"=w693:dbl, "Stats.TRA Position X"=w695:dbl[], "Stats.TRA PositionY"=w694:dbl[], "Stats.Stat Centriod X"=w722:dbl[], "Mean Centriod Y"=w721:dbl[], "Stats.Time"=w718:timestamp[])
        n309 = case shown="\"xpos\", Default" w696 {
          tunnel: w695 -> [w733 w741 w750 w758]
          tunnel: w694 -> [w730 w738 w748 w756]
          tunnel: w693 -> [w734 w742 w751 w759]
          tunnel: [w732 w740 w747 w755] -> w691
          tunnel: [w729 w737 w745 w753] -> w692
          frame "xpos", Default {
            n310 = Reverse 1D Array(array=w730) -> (reversed array=w731:dbl[])
            n311 = Reverse 1D Array(array=w733) -> (reversed array=w736:dbl[])
            n312 = Index Array(array=w731) -> (element=w729:dbl)  [unwired: 1 in]
            n313 = Index Array(array=w736) -> (element=w735:dbl)  [unwired: 1 in]
            n314 = Add(x=w735, y=w734) -> (x+y=w732:dbl)
          }
          frame "xneg" {
            n315 = Reverse 1D Array(array=w738) -> (reversed array=w739:dbl[])
            n316 = Reverse 1D Array(array=w741) -> (reversed array=w744:dbl[])
            n317 = Index Array(array=w739) -> (element=w737:dbl)  [unwired: 1 in]
            n318 = Index Array(array=w744) -> (element=w743:dbl)  [unwired: 1 in]
            n319 = Subtract(x=w743, y=w742) -> (x-y=w740:dbl)
          }
          frame "yneg" {
            n320 = Reverse 1D Array(array=w748) -> (reversed array=w749:dbl[])
            n321 = Reverse 1D Array(array=w750) -> (reversed array=w752:dbl[])
            n322 = Index Array(array=w749) -> (element=w746:dbl)  [unwired: 1 in]
            n323 = Index Array(array=w752) -> (element=w747:dbl)  [unwired: 1 in]
            n324 = Subtract(x=w746, y=w751) -> (x-y=w745:dbl)
          }
          frame "ypos" {
            n325 = Reverse 1D Array(array=w756) -> (reversed array=w757:dbl[])
            n326 = Reverse 1D Array(array=w758) -> (reversed array=w760:dbl[])
            n327 = Index Array(array=w757) -> (element=w754:dbl)  [unwired: 1 in]
            n328 = Index Array(array=w760) -> (element=w755:dbl)  [unwired: 1 in]
            n329 = Add(x=w754, y=w759) -> (x+y=w753:dbl)
          }
        }
        n330 = local read "Y offset"() -> (w719:dbl)
        n331 = local read "X offset"() -> (w720:dbl)
        n332 = Get Date/Time In Seconds() -> (seconds since 1Jan1904=w717:timestamp)
        n333 = Decrement(x=w698) -> (x-1=w697:i32)
        n334 = Build Array (concatenate)(w722, w720) -> (w723:dbl[])
        n335 = Build Array (concatenate)(w721, w719) -> (w701:dbl[])
        n336 = Array Size(array=w701) -> (size(s)=w700:i32)
        n337 = Quotient & Remainder(x=w700, y=w698) -> (x-y*floor(x/y)=w699:i32)  [unwired: 1 out]
        n338 = Build Array (concatenate)(w718, w717) -> (w716:timestamp[])
        n339 = Build Array (concatenate)(w695, w691) -> (w726:dbl[])
        n340 = Build Array (concatenate)(w694, w692) -> (w724:dbl[])
        n341 = Equal?(x=w699, y=w697) -> (x = y?=w704:bool)
        n342 = Bundle By Name(cluster=w725, "Stats.TRA Position X"=w726, "Stats.TRA PositionY"=w724, "Stats.Stat Centriod X"=w723, "Stats.Stat Centriod Y"=w701, "Stats.Time"=w716) -> (w715:T20)
        n343 = case shown="True" w704 {
          tunnel: w703 -> [w761 w764]
          tunnel: [w761 w762] -> w702
          frame False {
          }
          frame True {
            n344 = call <vilib>:"Add State(s) to Queue__jki_lib_state_machine.vi"("State(s) in (\"\")"=w764, "State(s) at Back (\"\")"="Save Stats" ("State(s) at Back (\"\")")) -> ("States Out"=w762:string)  [unwired: 13 in]
          }
        }
        n345 = Unbundle By Name(w715) -> ("Stats.Time"=w711:timestamp[], "Stats.Stat Centriod X"=w714:dbl[], "Stats.Stat Centriod Y"=w713:dbl[], "Stats.TRA Position X"=w712:dbl[], "Stats.TRA PositionY"=w710:dbl[])
        n346 = call <vilib>:"Add State(s) to Queue__jki_lib_state_machine.vi"("State(s) in (\"\")"=w702) -> ("States Out"=w728:string)  [unwired: 14 in]
        n347 = Bundle("Time"=w711, "Stat Centriod X"=w714) -> (w709:T23)  [unwired: 1 in]
        n348 = Bundle("Time"=w711, "Stat Centriod Y"=w713) -> (w708:T24)  [unwired: 1 in]
        n349 = Bundle("Time"=w711, "TRA Position X"=w712) -> (w707:T25)  [unwired: 1 in]
        n350 = Bundle("Time"=w711, "TRA PositionY"=w710) -> (w706:T26)  [unwired: 1 in]
        n351 = Build Array(w709, w708, w707, w706) -> (→"Stats":T27)
      }
      frame "Calibrate" {
        # "Your code here.\n(You can make a copy of, or modify, this frame)"
        n352 = Unbundle By Name(w776) -> ("RelativeMove.Axis 1.CW::2"=w769:refnum<vi>, "RelativeMove.Axis 1.CCW::2"=w768:refnum<vi>)
        n353 = control-ref of="RelativeSettings.Axis 1.Position::2"() -> (w767:refnum<vi>)
        n354 = Unbundle By Name(w775) -> ("beam detection para"=w771:T4)
        n355 = Decimal String To Number(string=w773) -> (number=w770:i32)  [unwired: 2 in, 1 out]
        n356 = Build Array(w767, w767) -> (w766:refnum<vi>[])
        n357 = Build Array(w769, w768) -> (w765:refnum<vi>[])
        n358 = call "CalibrateSingleAxis.vi"("Numeric"=w770, "beam detection para"=w771, "error in (no error)"=w774, "RelativeSettings.Axis 1"=w766, "RelativeMove.Axis 1"=w765, "Refnum in"=w772) -> ()  [unwired: 2 in, 4 out]
        n359 = call <vilib>:"Add State(s) to Queue__jki_lib_state_machine.vi"("State(s) in (\"\")"=w778) -> ("States Out"=w777:string)  [unwired: 14 in]
      }
      frame "New Category: 2" {
        # "Your code here.\n(You can make a copy of, or modify, this frame)"
        n360 = call <vilib>:"Add State(s) to Queue__jki_lib_state_machine.vi"("State(s) in (\"\")"=w782) -> ("States Out"=w781:string)  [unwired: 14 in]
      }
    }
    n361 = disable-structure shown="Disabled" {
      disable-tunnel: "ActiveMotorName::2" -> [w53 _]
      disable-tunnel: "ActiveMotor" -> [w50 _]
      frame Disabled {
        n362 = property on="ActiveMotor" class="Ring (strict)"() -> ("Strings []"=w49:string[])  [unwired: 2 in, 2 out]
        n363 = Index Array(array=w49, index=w50) -> (element=w51:string)
        n364 = Not Equal?(x=w53, y=w51) -> (x != y?=w52:bool)
        n365 = case shown="True" w52 {
          tunnel: w49 -> [_ w56]
          tunnel: w53 -> [_ w55]
          frame False {
          }
          frame True {
            n366 = Search 1D Array(1D array=w56, element=w55) -> (index of element=w54:i32)  [unwired: 1 in]
            n367 = property on="ActiveMotor" class="Ring (strict)"("Value"=w54) -> ()  [unwired: 2 in, 2 out]
          }
        }
      }
      frame Enabled {
      }
    }
  }
  n368 = control-ref of="This Application"() -> (w11:refnum<vi>)
  n369 = control-ref of="This VI"() -> (w15:refnum<vi>)
  n370 = Current VI's Menubar() -> (w14:refnum<k9>)
  n371 = call "supergui create stop queue.vi"() -> ("STOP Queue out"=w1:refnum<queue>)  [unwired: 11 in]
  n372 = call "GUI_Master_subvi_reentrant_queues.vi"("STOP Queue in"=w1, "This Application"=w11, "error in (no error)"=w12, "tcp data event"=w10, "Caller menu reference"=w14, "Caller VI ref"=w15) -> ("error out"=w23:errorcluster)  [unwired: 5 in]
  n373 = call <vilib>:"Clear Errors.vi"("error in (no error)"=w23) -> ("error out"=w21:errorcluster)  [unwired: 5 in, 1 out]
  n374 = call "IMAQ Dispose"("error in (no error)"=w21) -> ("error out"=w20:errorcluster)  [unwired: 5 in]
  n375 = call "IMAQ Dispose"("Image"=w16, "error in (no error)"=w20) -> ("error out"=→"error IO 2":errorcluster)  [unwired: 4 in]
